vi "MonoVu_exec window.vi"() -> ()   [LabVIEW 2020]
doc: "Sequence Program with the Message Handling Queue (MHQ) for the National High Magnetic Field Laboratory in Tallahassee, Florida. \nOnce you understand how the programs works, you should be able to modify this program easily. If you have any questions, contact Minseong Lee(ml10k@my.fsu.edu), who first made this program in June, 2015."
uses:
  <vilib>/printing/OpenHTMLReport.llb/Open HTML Report in Browser (String).vi
  <vilib>/Utility/NIReport.llb/NI_ReportGenerationCore.lvlib
panel:
  in  "error\ncheck":bool
  out "macro line":i32
  in  "loop stop":bool
  in  "looped command interval (ms)":u32=100
  in  "wait (ms)":u32
  in  "reset error indicator":bool
  out "Error/\nwarning?":bool
  in  "override command error":bool
  in  "platform":u16(ring) items=["Mac", "PC"]
  out "execution count":i32=1
  in  "sequence utility":bool=TRUE caption="seq\n utility"
  out "macro cmd no":i32=34
  in  "go to \ncurrent":bool
  in  "help":bool caption="Help"
  in  "Magnet PS":u16(ring) items=["Resistive Magnet", "SCM2", "SCM1", "Generic SC power supply", "PPMS"]
  out "Buffer Edit":string[](array[string])
  out "Path":path=path "/Users/Shared/NML Data Acquisition/Monovu/sequence templates/SystemABDE_typical.txt"
  out "Buffer History":string[](array[string])
  in  "NML Data Acquisition VI":string(combo)="NML Data Acquisition-New.vi"
  in  "Skip Button":bool caption="Skip"
  out "latest error":errorcluster={"status"=TRUE, "code"=1004, "source"="Open VI Reference in Get_Vi_Data.vi->WaitForAnyVI.vi->MonoVu.vi<APPEND>\nTo load a VI into memory with the Open VI Reference function, a path must be wired for the VI Path input.\n\nVI Name: <b>BLM_ManualControl.vi</b>"}
  in  "error in (no error)":errorcluster
  in  "New Button":bool caption="New"
  in  "Program Stop":bool caption="Program \nStop"
  out "Sequence Status":string="Idle"
  in  "Commands":string(tree)="Set Field"
  in  "Sequence":i32[](listbox)=[19]
  in  "Save Button":bool caption="Save"
  in  "Sequence_Stop":bool caption="Stop"
  in  "Pause Button":bool caption="Pause"
  in  "Run Sequence":bool caption="Run"
  in  "Save As Button":bool caption="Save As"
  out "Cursor Position":i32=19
  out "Current Line":i32
  in  "Open Button":bool caption="Open"
  # "Wait between each execution of command.\ne.g.  if the value is 10, and the command is \n'Wait for Temperature', it checks the temperature every 10 msec. It also forces pause between commands."
  # "(see logbook for previous errors)"
  # "(bypass command syntax error)"
  # "1. Each comand in the sequence line is executed repeatedly until a 'go to next line' command is issued by itself or interrupted by the user. \n2. 'go to next line' condition is defined in the VI for each command. \n\nNote\n(1) For commands with timed or conditioned wait, 'go to next line' command will be issued when the certain condition is met.\n(2) For non-wait command (send command to instruments or VI without waiting response), 'go to next line' is executed automatically.\n(3) For example, 'wait for temperature command' executes repeatedly until the temperature condition is met. The visa reference will be open and closed every time it is executed.\n** Exception: 'Wait for VI value' uses a loop to use the VI reference. The loop condition has to be programmatically reset for the user intervention (skip, pause, stop) accordingly."
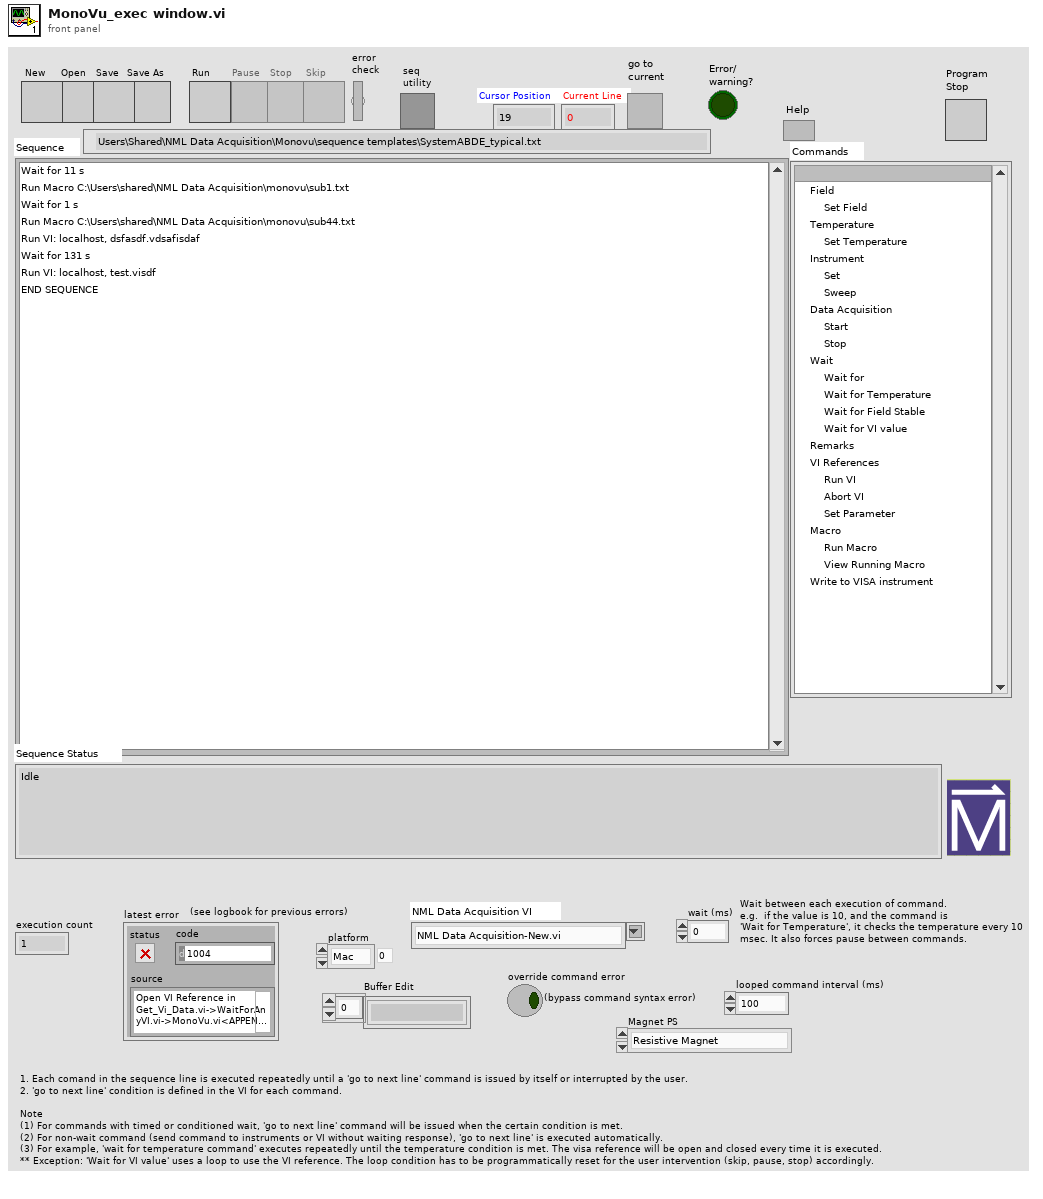
[diagram p1: front panel]
types:
  T1 = cluster{"Sequence_Run":refnum<vi>, "Sequence_Pause":refnum<vi>, "Sequence_Stop":refnum<vi>, "Sequence_Skip":refnum<vi>, "Program Stop":refnum<vi>, "Sequence":refnum<vi>, "NML Data Acquisition VI":refnum<vi>}
  T2 = cluster{"number of line":i32, "Signal":bool, "Command":string, "Sequence Reference":refnum<vi>, "Add or modification":bool}
  T3 = cluster{"No. of command":i32, "Parameters":string[], "Address":refnum<visa-resource-name>, "Boolean":bool, "No. of line":i32, "Initial Time":timestamp, "Current Time":timestamp, "Status":string, "Sequence Ref.":refnum<vi>, "Temp_Check":i32, "Sequence_History":string, "Subsequence":string[]}
  T4 = typedef "Command_Message.ctl" = cluster{"No. of command":i32, "Parameters":string[], "Address":refnum<visa-resource-name>, "Boolean":bool, "No. of line":i32, "Initial Time":timestamp, "Current Time":timestamp, "Status":string, "Sequence Ref.":refnum<vi>, "Temp check":i32, "Sequence_History":string, "Subsequence":string[]}
  T5 = typedef "Button_Reference.ctl" = cluster{"Sequence_Run":refnum<vi>, "Sequence_Pause":refnum<vi>, "Sequence_Stop":refnum<vi>, "Sequence_Skip":refnum<vi>, "Program Stop":refnum<vi>, "Sequence":refnum<vi>, "NML Data Acquisition VI":refnum<vi>}
  T6 = typedef "Command_Queue.ctl" = refnum<queue>
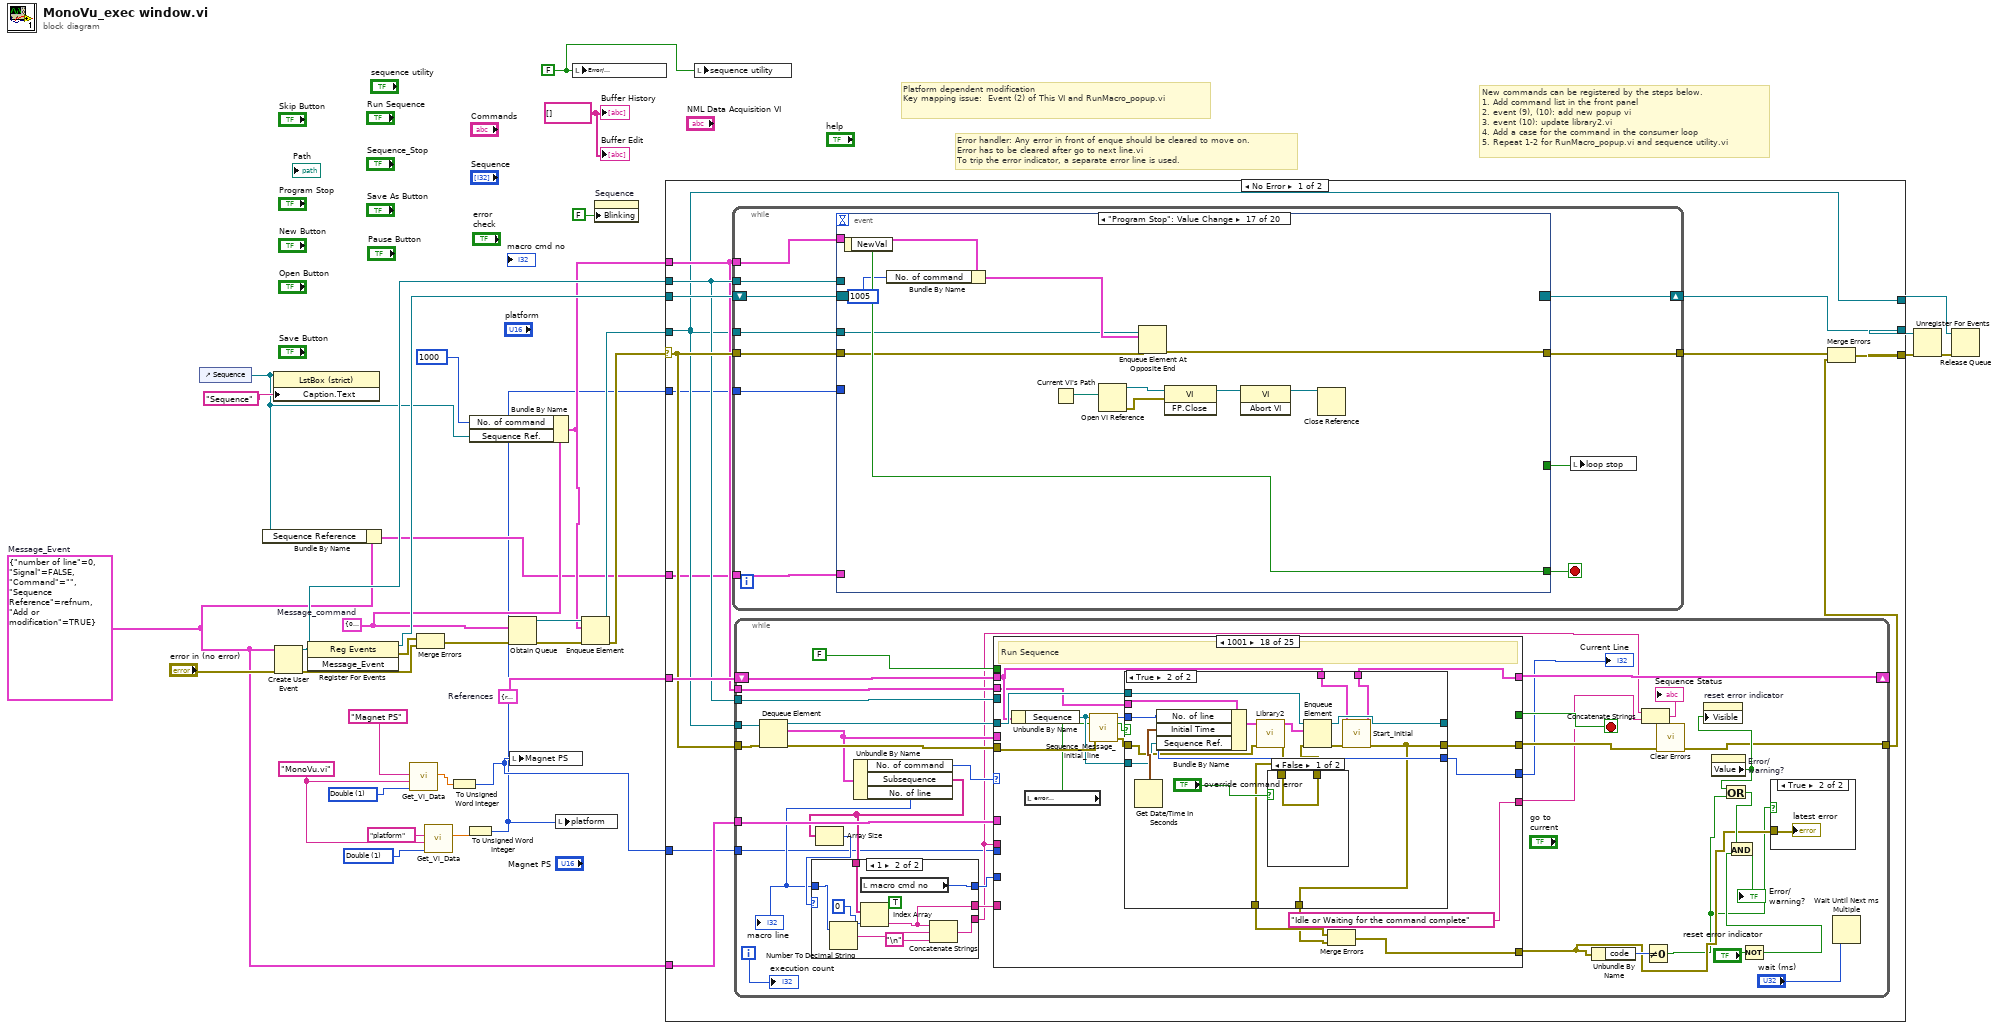
[diagram p0: block diagram]
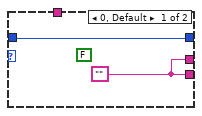
[diagram p3: hidden frame]
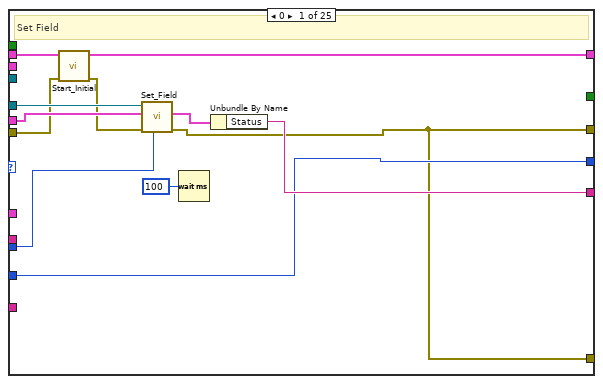
[diagram p4: hidden frame]
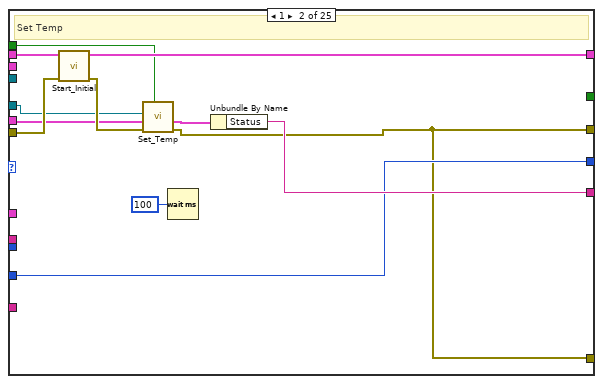
[diagram p5: hidden frame]
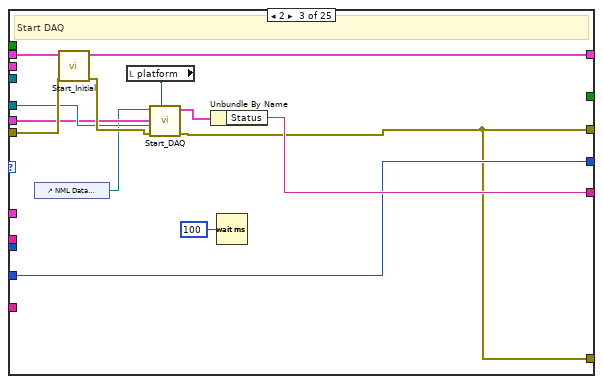
[diagram p6: hidden frame]
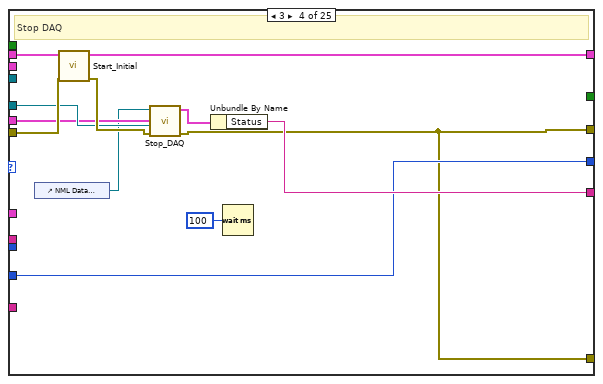
[diagram p7: hidden frame]
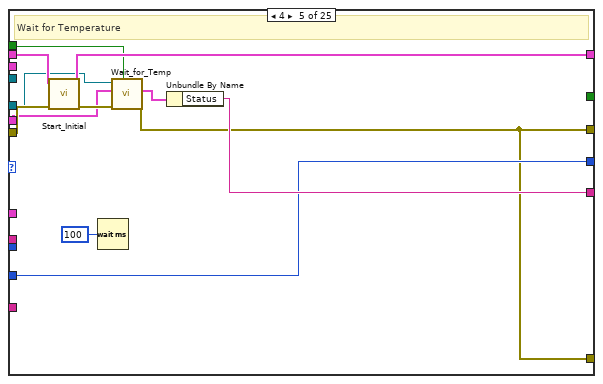
[diagram p8: hidden frame]
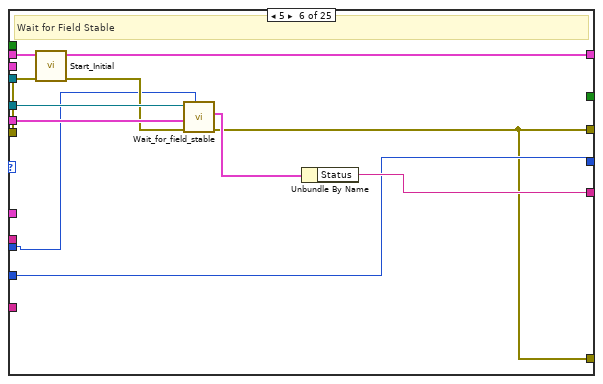
[diagram p9: hidden frame]
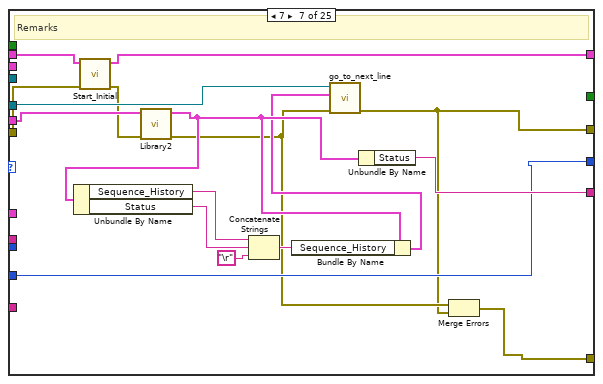
[diagram p10: hidden frame]
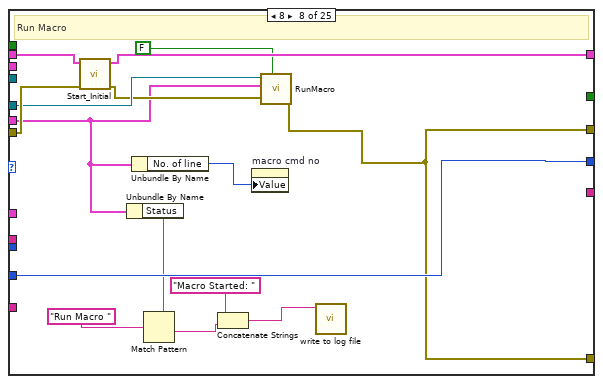
[diagram p11: hidden frame]
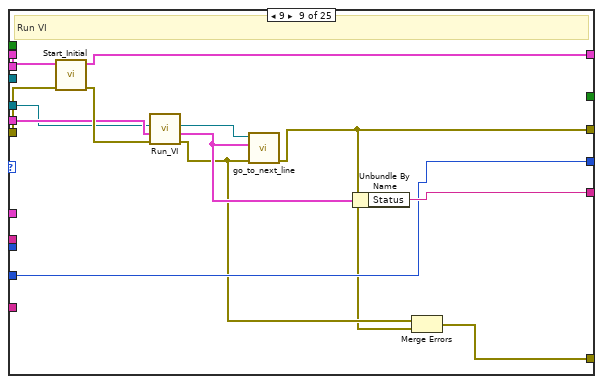
[diagram p12: hidden frame]
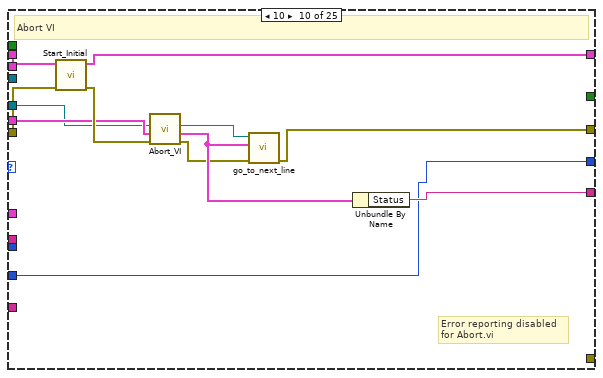
[diagram p13: hidden frame]
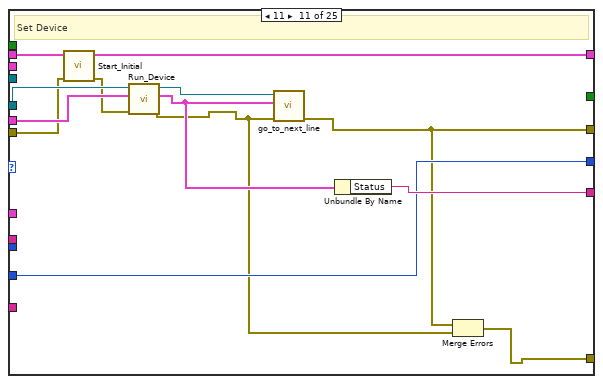
[diagram p14: hidden frame]
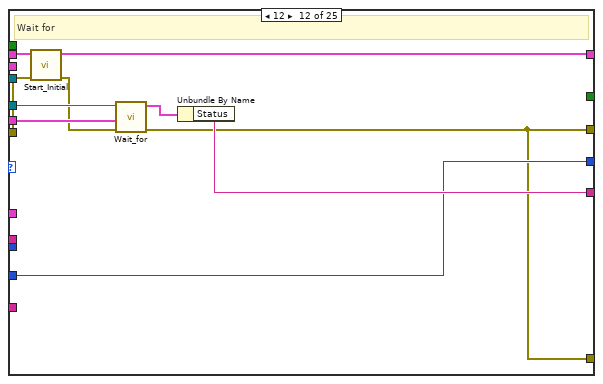
[diagram p15: hidden frame]
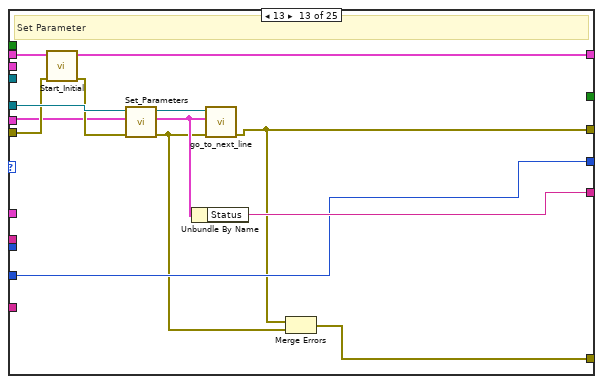
[diagram p16: hidden frame]
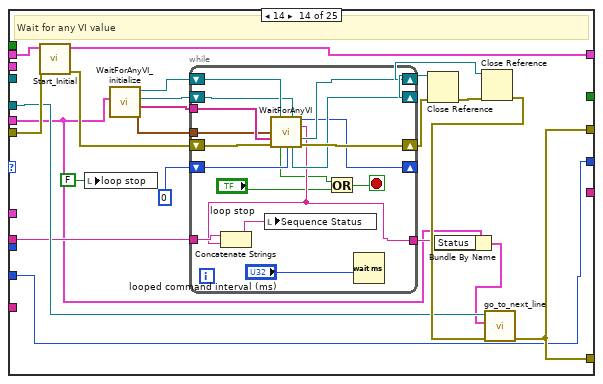
[diagram p17: hidden frame]
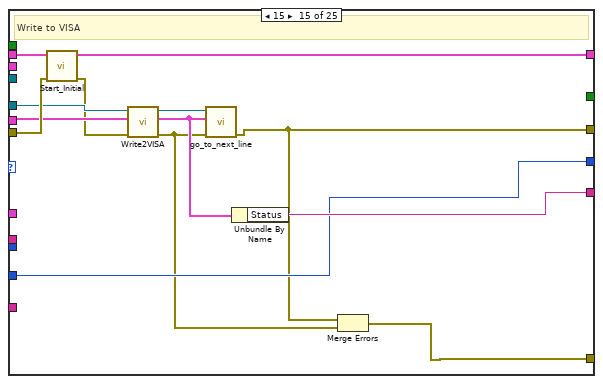
[diagram p18: hidden frame]
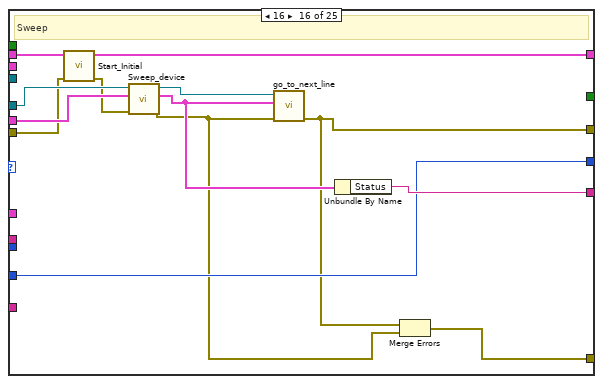
[diagram p19: hidden frame]
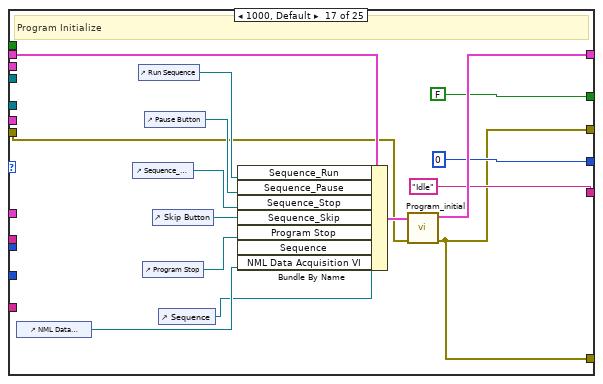
[diagram p20: hidden frame]
diagram:
  w7 = u16 1 items=["String", "Double", "Boolean", "Variant"] ("Data Type")
  w8 = u16 1 items=["String", "Double", "Boolean", "Variant"] ("Data Type")
  w6 = "MonoVu.vi" ("VI Name")
  w10 = FALSE ("Error?")
  w24 = T1 {"Sequence_Run"=refnum, "Sequence_Pause"=refnum, "Sequence_Stop"=refnum, "Sequence_Skip"=refnum, "Program Stop"=refnum, "Sequence"=refnum, "NML Data Acquisition VI"=refnum}  # References
  w12 = string[] []
  w18 = T2 {"number of line"=0, "Signal"=FALSE, "Command"="", "Sequence Reference"=refnum, "Add or modification"=TRUE}  # Message_Event
  w25 = T3 {"No. of command"=0, "Parameters"=[], "Address"="", "Boolean"=TRUE, "No. of line"=0, "Initial Time"=timestamp(0 s since 1904-01-01), "Current Time"=timestamp(0 s since 1904-01-01), "Status"="", "Sequence Ref."=refnum, "Temp_Check"=0, "Sequence_History"="", "Subsequence"=[]}  # Message_command
  # "Error handler: Any error in front of enque should be cleared to move on.\nError has to be cleared after go to next line.vi\nTo trip the error indicator, a separate error line is used."
  # "Platform dependent modification\nKey mapping issue:  Event (2) of This VI and RunMacro_popup.vi"
  # "New commands can be registered by the steps below.\n1. Add command list in the front panel\n2. event (9), (10): add new popup vi\n3. event (10): update library2.vi \n4. Add a case for the command in the consumer loop\n5. Repeat 1-2 for RunMacro_popup.vi and sequence utility.vi"
  n1 = control-ref of="Sequence"() -> (w13:refnum<vi>)
  n2 = Bundle By Name(cluster=w18, "Sequence Reference"=w13) -> (w17:T2)
  n3 = property class="LstBox (strict)"(reference=w13, "Caption.Text"="Sequence") -> ()  [unwired: 1 in, 2 out]
  n4 = Create User Event(user event datatype=w18, error in="error in (no error)") -> (user event=w30:refnum<user-event>, error out=w32:errorcluster)
  n5 = register-events(w30) -> (reference out=w34:refnum<event-registration>, error out=w31:errorcluster)  [unwired: 2 in]
  n6 = call "Get_Vi_Data.vi"("Data Type"=w8, "VI name"=w6, "Control Name"="Magnet PS") -> ("Data (Double)"=w4:dbl)  [unwired: 4 in, 4 out]
  n7 = Merge Errors(w31, w32) -> (w15:errorcluster)
  n8 = call "Get_Vi_Data.vi"("Data Type"=w7, "VI name"=w6, "Control Name"="platform") -> ("Data (Double)"=w3:dbl)  [unwired: 4 in, 4 out]
  n9 = To Unsigned Word Integer(number=w4) -> (unsigned 16bit integer=w2:u16)
  n10 = To Unsigned Word Integer(number=w3) -> (unsigned 16bit integer=w1:u16)
  n11 = Bundle By Name(cluster=w25, "No. of command"=1000, "Sequence Ref."=w13) -> (w23:T3)
  n12 = Obtain Queue(element data type=w25, error in (no error)=w15) -> (queue out=w29:refnum<queue>, error out=w27:errorcluster)  [unwired: 3 in, 1 out]
  n13 = local write "Magnet PS"(w2) -> ()
  n14 = local write "platform"(w1) -> ()
  n15 = local write "Error/\nwarning?"(w10) -> ()
  n16 = Enqueue Element(queue=w29, element=w23, error in (no error)=w27) -> (queue out=w28:refnum<queue>, error out=w26:errorcluster)  [unwired: 1 in, 1 out]
  n17 = property on="Sequence" class="LstBox (strict)"("Blinking"=FALSE) -> ()  [unwired: 2 in, 2 out]
  n18 = case shown="No Error" w26 {
    selector: w26 -> [w45 w1342]
    tunnel: w28 -> [w41 w1340]
    tunnel: [w47 w1342] -> w20
    tunnel: w30 -> [w44 _]
    tunnel: w34 -> [w48 w1341]
    tunnel: w24 -> [w46 _]
    tunnel: w23 -> [w42 _]
    tunnel: w18 -> [w43 _]
    tunnel: [w41 w1340] -> w22
    tunnel: [w39 w1341] -> w21
    tunnel: w17 -> [w37 _]
    tunnel: w1 -> [w36 _]
    tunnel: w2 -> [w35 _]
    frame No Error {
      n19 = while {
        tunnel: w41 -> [w486]
        tunnel: w44 -> [w485]
        tunnel: w45 -> [w484]
        tunnel: [w483] -> w40
        tunnel: w42 -> [w482]
        shift-right: [w481] -> w39
        shift-left: w48 -> [w488]
        tunnel: w37 -> [w480]
        tunnel: w36 -> [w479]
        stop <- w487 stop-if-true
        # "Event_Handler"
        n20 = event shown="[16] \"Program Stop\": Value Change" {
          selector: w488 -> [_ _ _ _ _ _ _ _ _ _ _ _ _ _ _ _ _ _ _ _]
          dyn-events: [_ _ _ _ _ _ _ _ _ _ _ _ _ _ _ _ _ _ _ _] -> w481
          timeout: _ -> [_ _ _ _ _ _ _ _ _ _ _ _ _ _ _ _ _ _ _ _]
          tunnel: [FALSE ("NewVal") FALSE ("NewVal") FALSE ("NewVal") FALSE ("NewVal") FALSE ("NewVal") FALSE ("NewVal") FALSE ("NewVal") FALSE ("NewVal") FALSE ("NewVal") FALSE ("NewVal") FALSE ("NewVal") FALSE ("NewVal") FALSE ("NewVal") FALSE ("NewVal") FALSE ("NewVal") FALSE ("NewVal") w1316 FALSE ("NewVal") TRUE ("NewVal") _] -> w487
          tunnel: w486 -> [w492 _ _ _ _ _ _ _ _ _ _ _ w1253 _ w1290 w1305 w1311 w1319 _ _]
          tunnel: w485 -> [w496 _ w680 w808 _ _ _ _ _ w983 w1112 _ _ _ _ _ _ _ _ _]
          tunnel: w484 -> [w495 w516 w681 w810 w840 w878 w892 w920 w947 w985 w1121 w1242 w1252 _ w1288 w1304 w1312 w1320 w1326 w1335]
          tunnel: [w491 w515 w679 w809 w839 w876 w891 w919 w946 w979 w1108 w1242 w1248 _ w1293 w1300 w1317 w1324 w1326 w1333] -> w483
          tunnel: w482 -> [w493 w514 _ _ _ _ _ _ _ _ w1123 _ w1251 _ w1294 w1303 w1315 w1323 _ _]
          tunnel: w480 -> [_ _ w682 w807 _ _ _ _ _ w977 w1113 _ _ _ _ _ _ _ _ _]
          tunnel: w479 -> [_ _ w676 _ _ _ _ _ _ w981 w1103 _ _ _ _ _ _ _ _ w1338]
          tunnel: [_ _ _ _ _ _ _ _ _ _ _ _ w1246 _ TRUE ("loop stop") TRUE ("loop stop") _ _ _ _] -> w478
          event "Run Sequence": Value Change {
            n21 = event-data() -> ("NewVal"=w494:bool)  [unwired: 1 in]
            n22 = case shown="True" w494 {
              tunnel: w496 -> [_ _]
              tunnel: w495 -> [w497 w501]
              tunnel: w493 -> [_ w504]
              tunnel: w492 -> [w498 w505]
              tunnel: [w498 w500] -> _
              tunnel: [w497 w499] -> w491
              frame False {
              }
              frame True {
                n23 = Bundle By Name(cluster=w504, "No. of command"=1001) -> (w502:T3)
                n24 = Enqueue Element At Opposite End(queue=w505, element=w502, error in (no error)=w501) -> (queue out=w500:refnum<queue>, error out=w499:errorcluster)  [unwired: 1 in, 1 out]
              }
            }
            n25 = call "write to log file.vi"("input"="Run button pressed") -> ()  [unwired: 9 in, 1 out]
          }
          event User Event {
            n26 = event-data() -> ("number of line"=w513:i32, "Command"=w507:string, "Signal"=w511:bool, "Sequence Reference"=w510:refnum<vi>, "Add or modification"=w509:bool)  [unwired: 1 in]
            n27 = local read "Buffer History"() -> (w508:string[])
            n28 = local read "Buffer Edit"() -> (w506:string[])
            n29 = case shown="\"Undo\"" w507 {
              selector: w507 -> [_ _ _ _ _ w632]
              tunnel: w516 -> [w520 w552 w584 w607 w630 w640]
              tunnel: [w518 w543 w575 w603 w616 w639] -> w515
              tunnel: w514 -> [_ _ _ _ _ w638]
              tunnel: w513 -> [_ _ _ _ _ w637]
              tunnel: w511 -> [_ _ _ _ _ w636]
              tunnel: w510 -> [w517 w553 w585 w608 w631 w635]
              tunnel: w509 -> [_ _ _ _ _ w634]
              tunnel: w508 -> [w519 w548 w580 _ w622 w633]
              tunnel: w506 -> [_ _ _ _ w625 _]
              frame "Undo" {
                n30 = Index Array(array=w519, index=0) -> (element=w527:string)
                n31 = Unflatten From String(type=w519, binary string=w527, error in (no error)=w520) -> (value=w526:string[], error out=w525:errorcluster)  [unwired: 2 in, 1 out]
                n32 = property on="Property Node" class="LstBox (strict)"(reference=w517, error in=w525, "Item Names"=w526) -> (error out=w521:errorcluster)  [unwired: 1 out]
                n33 = Delete From Array(array=w519, length=1, index=0) -> (array with subset deleted=w522:string[])  [unwired: 1 out]
                n34 = property on="Buffer History" class="Arr (strict)"(error in=w521, "Val(Sgnl)"=w522) -> (error out=w518:errorcluster)  [unwired: 1 in, 1 out]
              }
              frame "Cut" {
                n35 = property on="Property Node" class="LstBox (strict)"(reference=w553, error in=w552) -> (reference out=w550:refnum<vi>, error out=w549:errorcluster, "Item Names"=w533:string[], "Value"=w529:i32[])
                n36 = Array Size(array=w529) -> (size(s)=w541:i32)
                n37 = Index Array(array=w529, index=0) -> (element=w540:i32)
                n38 = Delete From Array(array=w533, length=w541, index=w540) -> (deleted portion=w531:string[], array with subset deleted=w534:string[])
                n39 = Array Size(array=w531) -> (size(s)=w539:i32)
                n40 = Decrement(x=w539) -> (x-1=w538:i32)
                n41 = Index Array(array=w531, index=w538) -> (element=w536:string)
                n42 = Equal?(x=w536, y="END SEQUENCE") -> (x = y?=w535:bool)
                n43 = case shown="True" w535 {
                  tunnel: w533 -> [_ w561]
                  tunnel: w541 -> [_ w560]
                  tunnel: w540 -> [_ w558]
                  tunnel: [w555 w557] -> w532
                  tunnel: w534 -> [w555 _]
                  tunnel: w531 -> [w554 _]
                  tunnel: [w554 w556] -> w530
                  frame False {
                  }
                  frame True {
                    n44 = Decrement(x=w560) -> (x-1=w559:i32)
                    n45 = Delete From Array(array=w561, length=w559, index=w558) -> (deleted portion=w556:string[], array with subset deleted=w557:string[])
                  }
                }
                n46 = Flatten To String(anything=w532, error in (no error)=w549) -> (data string=w546:string, error out=w545:errorcluster)  [unwired: 2 in, 1 out]
                n47 = property on="Property Node" class="LstBox (strict)"(reference=w550, error in=w545, "Item Names"=w532, "Val(Sgnl)"=w529) -> (error out=w544:errorcluster)  [unwired: 1 out]
                n48 = Insert Into Array(array=w548, index=0, new element=w546) -> (w542:string[])
                n49 = property on="Buffer History" class="Arr (strict)"(error in=w544, "Val(Sgnl)"=w542) -> (error out=w543:errorcluster)  [unwired: 1 in, 1 out]
                n50 = local write "Buffer Edit"(w530) -> ()
              }
              frame "Delete" {
                n51 = property on="Property Node" class="LstBox (strict)"(reference=w585, error in=w584) -> (reference out=w582:refnum<vi>, error out=w581:errorcluster, "Item Names"=w567:string[], "Value"=w562:i32[])
                n52 = Array Size(array=w562) -> (size(s)=w566:i32)
                n53 = Index Array(array=w562, index=0) -> (element=w565:i32)
                n54 = Delete From Array(array=w567, length=w566, index=w565) -> (deleted portion=w573:string[], array with subset deleted=w564:string[])
                n55 = Array Size(array=w573) -> (size(s)=w569:i32)
                n56 = Decrement(x=w569) -> (x-1=w568:i32)
                n57 = Index Array(array=w573, index=w568) -> (element=w572:string)
                n58 = Equal?(x=w572, y="END SEQUENCE") -> (x = y?=w570:bool)
                n59 = case shown="True" w570 {
                  tunnel: w567 -> [_ w591]
                  tunnel: w566 -> [_ w590]
                  tunnel: w565 -> [_ w588]
                  tunnel: [w586 w587] -> w563
                  tunnel: w564 -> [w586 _]
                  frame False {
                  }
                  frame True {
                    n60 = Decrement(x=w590) -> (x-1=w589:i32)
                    n61 = Delete From Array(array=w591, length=w589, index=w588) -> (array with subset deleted=w587:string[])  [unwired: 1 out]
                  }
                }
                n62 = Flatten To String(anything=w563, error in (no error)=w581) -> (data string=w578:string, error out=w577:errorcluster)  [unwired: 2 in, 1 out]
                n63 = property on="Property Node" class="LstBox (strict)"(reference=w582, error in=w577, "Item Names"=w563, "Val(Sgnl)"=w562) -> (error out=w576:errorcluster)  [unwired: 1 out]
                n64 = Insert Into Array(array=w580, index=0, new element=w578) -> (w574:string[])
                n65 = property on="Buffer History" class="Arr (strict)"(error in=w576, "Val(Sgnl)"=w574) -> (error out=w575:errorcluster)  [unwired: 1 in, 1 out]
              }
              frame "Copy" {
                n66 = property on="Property Node" class="LstBox (strict)"(reference=w608, error in=w607) -> (reference out=w605:refnum<vi>, error out=w604:errorcluster, "Item Names"=w593:string[], "Value"=w592:i32[])
                n67 = Array Size(array=w592) -> (size(s)=w597:i32)
                n68 = Index Array(array=w592, index=0) -> (element=w596:i32)
                n69 = Array Subset(array=w593, index=w596, length=w597) -> (w595:string[])
                n70 = Array Size(array=w595) -> (size(s)=w602:i32)
                n71 = Decrement(x=w602) -> (x-1=w601:i32)
                n72 = property on="Property Node" class="LstBox (strict)"(reference=w605, error in=w604, "Item Names"=w593, "Val(Sgnl)"=w592) -> (error out=w603:errorcluster)  [unwired: 1 out]
                n73 = Index Array(array=w595, index=w601) -> (element=w600:string)
                n74 = Equal?(x=w600, y="END SEQUENCE") -> (x = y?=w598:bool)
                n75 = case shown="True" w598 {
                  tunnel: w597 -> [_ w614]
                  tunnel: w596 -> [_ w612]
                  tunnel: [w609 w610] -> w594
                  tunnel: w595 -> [w609 _]
                  tunnel: w593 -> [_ w611]
                  frame False {
                  }
                  frame True {
                    n76 = Decrement(x=w614) -> (x-1=w613:i32)
                    n77 = Delete From Array(array=w611, length=w613, index=w612) -> (deleted portion=w610:string[])  [unwired: 1 out]
                  }
                }
                n78 = local write "Buffer Edit"(w594) -> ()
              }
              frame "Paste" {
                n79 = property on="Property Node" class="LstBox (strict)"(reference=w631, error in=w630) -> (reference out=w628:refnum<vi>, error out=w619:errorcluster, "Item Names"=w626:string[], "Value"=w615:i32[])
                n80 = Index Array(array=w615, index=0) -> (element=w627:i32)
                n81 = Insert Into Array(array=w626, index=w627, new element=w625) -> (w623:string[])
                n82 = Flatten To String(anything=w623, error in (no error)=w619) -> (data string=w624:string, error out=w618:errorcluster)  [unwired: 2 in, 1 out]
                n83 = property on="Property Node" class="LstBox (strict)"(reference=w628, error in=w618, "Item Names"=w623, "Val(Sgnl)"=w615) -> (error out=w617:errorcluster)  [unwired: 1 out]
                n84 = Insert Into Array(array=w622, index=0, new element=w624) -> (w620:string[])
                n85 = property on="Buffer History" class="Arr (strict)"(error in=w617, "Val(Sgnl)"=w620) -> (error out=w616:errorcluster)  [unwired: 1 in, 1 out]
              }
              frame Default {
                n86 = case shown="True" w634 {
                  tunnel: w640 -> [w657 w674]
                  tunnel: [w642 w659] -> w639
                  tunnel: w638 -> [_ _]
                  tunnel: w637 -> [_ _]
                  tunnel: w636 -> [_ _]
                  tunnel: w635 -> [w656 w673]
                  tunnel: w632 -> [w655 w672]
                  tunnel: w633 -> [w654 w671]
                  frame True {
                    n87 = property class="LstBox (strict)"(reference=w656, error in=w657) -> (reference out=w651:refnum<vi>, error out=w646:errorcluster, "Item Names"=w648:string[], "Value"=w641:i32[])
                    n88 = Index Array(array=w641, index=0) -> (element=w652:i32)
                    n89 = Flatten To String(anything=w648, error in (no error)=w646) -> (data string=w649:string, error out=w647:errorcluster)  [unwired: 2 in, 1 out]
                    n90 = Insert Into Array(array=w648, index=w652, new element=w655) -> (w650:string[])
                    n91 = property class="LstBox (strict)"(reference=w651, error in=w647, "Item Names"=w650, "Value"=w641) -> (error out=w643:errorcluster)  [unwired: 1 out]
                    n92 = Insert Into Array(array=w654, index=0, new element=w649) -> (w644:string[])
                    n93 = property on="Buffer History" class="Arr (strict)"(error in=w643, "Val(Sgnl)"=w644) -> (error out=w642:errorcluster)  [unwired: 1 in, 1 out]
                  }
                  frame False {
                    n94 = property class="LstBox (strict)"(reference=w673, error in=w674) -> (reference out=w668:refnum<vi>, error out=w664:errorcluster, "Item Names"=w665:string[], "Value"=w658:i32[])
                    n95 = Index Array(array=w658, index=0) -> (element=w669:i32)
                    n96 = Flatten To String(anything=w665, error in (no error)=w664) -> (data string=w667:string, error out=w663:errorcluster)  [unwired: 2 in, 1 out]
                    n97 = Replace Array Subset(array=w665, new element=w672, index=w669) -> (w666:string[])
                    n98 = property class="LstBox (strict)"(reference=w668, error in=w663, "Item Names"=w666) -> (error out=w661:errorcluster)  [unwired: 1 out]
                    n99 = Insert Into Array(array=w671, index=0, new element=w667) -> (w660:string[])
                    n100 = property on="Buffer History" class="Arr (strict)"(error in=w661, "Val(Sgnl)"=w660) -> (error out=w659:errorcluster)  [unwired: 1 in, 1 out]
                  }
                }
              }
            }
          }
          event "Sequence": Key Down {
            # "PC:\nDelete:  83\nundo: 44\ncut: 45\ncopy: 46\npaste: 47"
            # "Mac:\nDelete:  117\nundo: 6\ncut: 7\ncopy: 8\npaste: 9"
            n101 = event-data() -> ("ScanCode"=w683:i16, "PlatMods.Ctrl"=w677:bool, "PlatMods.Shift"=w675:bool)  [unwired: 1 in]
            n102 = case shown="0, Default" w676 {
              tunnel: w683 -> [w689 w750]
              tunnel: w682 -> [w688 w749]
              tunnel: w681 -> [w687 w748]
              tunnel: w680 -> [w686 w747]
              tunnel: [w685 w746] -> w679
              tunnel: w677 -> [_ w745]
              tunnel: w675 -> [w684 _]
              frame 1 {
                n103 = case shown="0, Default" w689 {
                  tunnel: w688 -> [_ w695 w698 w710 w722 w734]
                  tunnel: w687 -> [w690 w693 w700 w712 w724 w736]
                  tunnel: w686 -> [_ w692 w697 w709 w721 w733]
                  tunnel: [w690 w691 w699 w711 w723 w735] -> w685
                  tunnel: w684 -> [_ _ w701 w713 w725 w737]
                  frame 0, Default {
                  }
                  frame 83 {
                    n104 = Bundle By Name(cluster=w695, "Command"="Delete") -> (w694:T2)
                    n105 = Generate User Event(user event=w692, event data cluster=w694, error in=w693) -> (error out=w691:errorcluster)  [unwired: 1 in, 1 out]
                  }
                  frame 44 {
                    n106 = case shown="True" w701 {
                      tunnel: w700 -> [w702 w704]
                      tunnel: [w702 w706] -> w699
                      tunnel: w698 -> [_ w705]
                      tunnel: w697 -> [_ w703]
                      frame False {
                      }
                      frame True {
                        n107 = Bundle By Name(cluster=w705, "Command"="Undo") -> (w707:T2)
                        n108 = Generate User Event(user event=w703, event data cluster=w707, error in=w704) -> (error out=w706:errorcluster)  [unwired: 1 in, 1 out]
                      }
                    }
                  }
                  frame 45 {
                    n109 = case shown="True" w713 {
                      tunnel: w712 -> [w714 w716]
                      tunnel: [w714 w718] -> w711
                      tunnel: w710 -> [_ w717]
                      tunnel: w709 -> [_ w715]
                      frame False {
                      }
                      frame True {
                        n110 = Bundle By Name(cluster=w717, "Command"="Cut") -> (w719:T2)
                        n111 = Generate User Event(user event=w715, event data cluster=w719, error in=w716) -> (error out=w718:errorcluster)  [unwired: 1 in, 1 out]
                      }
                    }
                  }
                  frame 46 {
                    n112 = case shown="True" w725 {
                      tunnel: w724 -> [w726 w728]
                      tunnel: [w726 w730] -> w723
                      tunnel: w722 -> [_ w729]
                      tunnel: w721 -> [_ w727]
                      frame False {
                      }
                      frame True {
                        n113 = Bundle By Name(cluster=w729, "Command"="Copy") -> (w731:T2)
                        n114 = Generate User Event(user event=w727, event data cluster=w731, error in=w728) -> (error out=w730:errorcluster)  [unwired: 1 in, 1 out]
                      }
                    }
                  }
                  frame 47 {
                    n115 = case shown="True" w737 {
                      tunnel: w736 -> [w738 w740]
                      tunnel: [w738 w742] -> w735
                      tunnel: w734 -> [_ w741]
                      tunnel: w733 -> [_ w739]
                      frame False {
                      }
                      frame True {
                        n116 = Bundle By Name(cluster=w741, "Command"="Paste") -> (w743:T2)
                        n117 = Generate User Event(user event=w739, event data cluster=w743, error in=w740) -> (error out=w742:errorcluster)  [unwired: 1 in, 1 out]
                      }
                    }
                  }
                }
              }
              frame 0, Default {
                n118 = case shown="0, Default" w750 {
                  tunnel: w749 -> [_ w756 w759 w771 w783 w795]
                  tunnel: w748 -> [w751 w754 w761 w773 w785 w797]
                  tunnel: w747 -> [_ w753 w758 w770 w782 w794]
                  tunnel: [w751 w752 w760 w772 w784 w796] -> w746
                  tunnel: w745 -> [_ _ w762 w774 w786 w798]
                  frame 0, Default {
                  }
                  frame 117 {
                    n119 = Bundle By Name(cluster=w756, "Command"="Delete") -> (w755:T2)
                    n120 = Generate User Event(user event=w753, event data cluster=w755, error in=w754) -> (error out=w752:errorcluster)  [unwired: 1 in, 1 out]
                  }
                  frame 6 {
                    n121 = case shown="True" w762 {
                      tunnel: w761 -> [w763 w765]
                      tunnel: [w763 w767] -> w760
                      tunnel: w759 -> [_ w766]
                      tunnel: w758 -> [_ w764]
                      frame False {
                      }
                      frame True {
                        n122 = Bundle By Name(cluster=w766, "Command"="Undo") -> (w768:T2)
                        n123 = Generate User Event(user event=w764, event data cluster=w768, error in=w765) -> (error out=w767:errorcluster)  [unwired: 1 in, 1 out]
                      }
                    }
                  }
                  frame 7 {
                    n124 = case shown="True" w774 {
                      tunnel: w773 -> [w775 w777]
                      tunnel: [w775 w779] -> w772
                      tunnel: w771 -> [_ w778]
                      tunnel: w770 -> [_ w776]
                      frame False {
                      }
                      frame True {
                        n125 = Bundle By Name(cluster=w778, "Command"="Cut") -> (w780:T2)
                        n126 = Generate User Event(user event=w776, event data cluster=w780, error in=w777) -> (error out=w779:errorcluster)  [unwired: 1 in, 1 out]
                      }
                    }
                  }
                  frame 8 {
                    n127 = case shown="True" w786 {
                      tunnel: w785 -> [w787 w789]
                      tunnel: [w787 w791] -> w784
                      tunnel: w783 -> [_ w790]
                      tunnel: w782 -> [_ w788]
                      frame False {
                      }
                      frame True {
                        n128 = Bundle By Name(cluster=w790, "Command"="Copy") -> (w792:T2)
                        n129 = Generate User Event(user event=w788, event data cluster=w792, error in=w789) -> (error out=w791:errorcluster)  [unwired: 1 in, 1 out]
                      }
                    }
                  }
                  frame 9 {
                    n130 = case shown="True" w798 {
                      tunnel: w797 -> [w799 w801]
                      tunnel: [w799 w803] -> w796
                      tunnel: w795 -> [_ w802]
                      tunnel: w794 -> [_ w800]
                      frame False {
                      }
                      frame True {
                        n131 = Bundle By Name(cluster=w802, "Command"="Paste") -> (w804:T2)
                        n132 = Generate User Event(user event=w800, event data cluster=w804, error in=w801) -> (error out=w803:errorcluster)  [unwired: 1 in, 1 out]
                      }
                    }
                  }
                }
              }
            }
          }
          event "Sequence": Shortcut Menu Selection (User) {
            n133 = event-data() -> ("ItemTag"=w811:string)  [unwired: 1 in]
            n134 = case shown="\"Paste\"" w811 {
              selector: w811 -> [_ w816 w822 w828 w834]
              tunnel: w810 -> [w812 w814 w820 w826 w832]
              tunnel: [w812 w813 w819 w825 w831] -> w809
              tunnel: w808 -> [_ w818 w824 w830 w836]
              tunnel: w807 -> [_ w817 w823 w829 w835]
              frame Default {
              }
              frame "Undo" {
                n135 = Bundle By Name(cluster=w817, "Command"=w816) -> (w815:T2)
                n136 = Generate User Event(user event=w818, event data cluster=w815, error in=w814) -> (error out=w813:errorcluster)  [unwired: 1 in, 1 out]
              }
              frame "Cut" {
                n137 = Bundle By Name(cluster=w823, "Command"=w822) -> (w821:T2)
                n138 = Generate User Event(user event=w824, event data cluster=w821, error in=w820) -> (error out=w819:errorcluster)  [unwired: 1 in, 1 out]
              }
              frame "Copy" {
                n139 = Bundle By Name(cluster=w829, "Command"=w828) -> (w827:T2)
                n140 = Generate User Event(user event=w830, event data cluster=w827, error in=w826) -> (error out=w825:errorcluster)  [unwired: 1 in, 1 out]
              }
              frame "Paste" {
                n141 = Bundle By Name(cluster=w835, "Command"=w834) -> (w833:T2)
                n142 = Generate User Event(user event=w836, event data cluster=w833, error in=w832) -> (error out=w831:errorcluster)  [unwired: 1 in, 1 out]
              }
            }
          }
          event "New Button": Value Change {
            n143 = event-data() -> ("NewVal"=w841:bool, "CtlRef"=w838:refnum<vi>)  [unwired: 1 in]
            n144 = case shown="True" w841 {
              tunnel: w840 -> [w842 w858]
              tunnel: [w842 w850] -> w839
              tunnel: w838 -> [_ w853]
              frame False {
              }
              frame True {
                n145 = property on="Sequence" class="LstBox (strict)"(error in=w858) -> (error out=w849:errorcluster, "Caption.Text"=w857:string, "Item Names"=w854:string[])  [unwired: 1 in, 1 out]
                n146 = property on="Buffer History" class="Arr (strict)"(error in=w849) -> (error out=w848:errorcluster, "Value"=w847:string[])  [unwired: 1 in, 1 out]
                n147 = Equal?(x=w857, y="Sequence*") -> (x = y?=w855:bool)
                n148 = case shown="False" w855 {
                  tunnel: w848 -> [w863 w874]
                  tunnel: w854 -> [_ w875]
                  tunnel: [w864 w869] -> w846
                  tunnel: w853 -> [w862 w868]
                  tunnel: [w862 w868] -> w852
                  tunnel: w847 -> [_ w866]
                  tunnel: [string[] [] ("Buffer out") w865] -> w844
                  frame False {
                    n149 = property on="Sequence" class="LstBox (strict)"(error in=w863, "Item Names"=string[] ["END SEQUENCE"], "Caption.Text"="Sequence") -> (error out=w864:errorcluster)  [unwired: 1 in, 1 out]
                  }
                  frame True {
                    n150 = property on="Path" class="Path"(error in=w874) -> (error out=w873:errorcluster, "Value"=w872:path)  [unwired: 1 in, 1 out]
                    n151 = call "New_File.vi"("error in (no error)"=w873, "Path"=w872, "Buffer in"=w866, "Sequence in"=w875) -> ("error out"=w871:errorcluster, "Sequence Caption"=w867:string, "Buffer out"=w865:string[], "Sequence_out"=w870:string[])  [unwired: 4 in]
                    n152 = property on="Sequence" class="LstBox (strict)"(error in=w871, "Item Names"=w870, "Caption.Text"=w867) -> (error out=w869:errorcluster)  [unwired: 1 in, 1 out]
                  }
                }
                n153 = property on="Buffer History" class="Arr (strict)"(error in=w846, "Value"=w844) -> (error out=w845:errorcluster)  [unwired: 1 in, 1 out]
                n154 = property class="Bool (strict)"(reference=w852, error in=w845, "Value"=FALSE) -> (error out=w850:errorcluster)  [unwired: 1 out]
                n155 = property on="Sequence" class="LstBox (strict)"("Top Row"=0) -> ()  [unwired: 2 in, 2 out]
              }
            }
          }
          event "Buffer History": Value Change {
            n156 = event-data() -> ("NewVal"=w882:string[])  [unwired: 1 in]
            n157 = Array Size(array=w882) -> (size(s)=w881:i32)
            n158 = Equal?(x=w881, y=0) -> (x = y?=w879:bool)
            n159 = case shown="False" w879 {
              tunnel: w878 -> [w884 w887]
              tunnel: [w883 w886] -> w876
              frame True {
                n160 = property on="Sequence" class="LstBox (strict)"(error in=w884, "Caption.Text"="Sequence") -> (error out=w883:errorcluster)  [unwired: 1 in, 1 out]
              }
              frame False {
                n161 = property on="Sequence" class="LstBox (strict)"(error in=w887, "Caption.Text"="Sequence*") -> (error out=w886:errorcluster)  [unwired: 1 in, 1 out]
              }
            }
          }
          event "Open Button": Value Change {
            n162 = event-data() -> ("NewVal"=w893:bool, "CtlRef"=w890:refnum<vi>)  [unwired: 1 in]
            n163 = case shown="True" w893 {
              tunnel: w892 -> [w894 w916]
              tunnel: [w894 w897] -> w891
              tunnel: w890 -> [_ w900]
              frame False {
              }
              frame True {
                n164 = property on="Sequence" class="LstBox (strict)"(error in=w916) -> (error out=w912:errorcluster, "Caption.Text"=w914:string, "Item Names"=w913:string[])  [unwired: 1 in, 1 out]
                n165 = Equal?(x=w914, y="Sequence*") -> (x = y?=w901:bool)
                n166 = property on="Buffer History" class="Arr (strict)"(error in=w912) -> (error out=w910:errorcluster, "Value"=w911:string[])  [unwired: 1 in, 1 out]
                n167 = property on="Path" class="Path"(error in=w910) -> (error out=w908:errorcluster, "Value"=w909:path)  [unwired: 1 in, 1 out]
                n168 = call "Open_File.vi"("Message?"=w901, "Path in"=w909, "error in (no error)"=w908, "Sequence in"=w913, "Buffer in"=w911, "Sequence Caption in"=w914) -> ("error out"=w896:errorcluster, "Sequence out"=w906:string[], "Buffer out"=w904:string[], "Sequence Caption out"=w907:string, "Path out"=w902:path, "top row"=w895:i32)
                n169 = property on="Sequence" class="LstBox (strict)"("Top Row"=w895) -> ()  [unwired: 2 in, 2 out]
                n170 = property on="Sequence" class="LstBox (strict)"(error in=w896, "Item Names"=w906, "Caption.Text"=w907) -> (error out=w905:errorcluster)  [unwired: 1 in, 1 out]
                n171 = property on="Buffer History" class="Arr (strict)"(error in=w905, "Value"=w904) -> (error out=w903:errorcluster)  [unwired: 1 in, 1 out]
                n172 = property on="Path" class="Path"(error in=w903, "Value"=w902) -> (error out=w899:errorcluster)  [unwired: 1 in, 1 out]
                n173 = property class="Bool (strict)"(reference=w900, error in=w899, "Value"=FALSE) -> (error out=w897:errorcluster)  [unwired: 1 out]
              }
            }
          }
          event "Save Button": Value Change {
            n174 = event-data() -> ("NewVal"=w921:bool, "CtlRef"=w918:refnum<vi>)  [unwired: 1 in]
            n175 = case shown="True" w921 {
              tunnel: w920 -> [w922 w939]
              tunnel: [w922 w923] -> w919
              tunnel: w918 -> [_ w926]
              frame False {
              }
              frame True {
                n176 = property on="Path" class="Path"(error in=w939) -> (error out=w938:errorcluster, "Value"=w941:path)  [unwired: 1 in, 1 out]
                n177 = Not Equal?(x=path "", y=w941) -> (x != y?=w942:bool)
                n178 = property on="Buffer History" class="Arr (strict)"(error in=w938) -> (error out=w937:errorcluster, "Value"=w940:string[])  [unwired: 1 in, 1 out]
                n179 = property on="Sequence" class="LstBox (strict)"(error in=w937) -> (error out=w936:errorcluster, "Item Names"=w935:string[], "Caption.Text"=w934:string)  [unwired: 1 in, 1 out]
                n180 = call "Save_File.vi"("Sequence caption in"=w934, "Path?"=w942, "error in (no error)"=w936, "Sequence in"=w935, "Buffer in"=w940, "Path in"=w941) -> ("error out"=w933:errorcluster, "Sequence out"=w929:string[], "Buffer out"=w931:string[], "Path out"=w927:path, "Sequence caption out"=w930:string)  [unwired: 1 in]
                n181 = property on="Buffer History" class="Arr (strict)"(error in=w933, "Value"=w931) -> (error out=w932:errorcluster)  [unwired: 1 in, 1 out]
                n182 = property on="Sequence" class="LstBox (strict)"(error in=w932, "Item Names"=w929, "Caption.Text"=w930) -> (error out=w928:errorcluster)  [unwired: 1 in, 1 out]
                n183 = property on="Path" class="Path"(error in=w928, "Value"=w927) -> (error out=w925:errorcluster)  [unwired: 1 in, 1 out]
                n184 = property class="Bool (strict)"(reference=w926, error in=w925, "Value"=FALSE) -> (error out=w923:errorcluster)  [unwired: 1 out]
              }
            }
          }
          event "Save As Button": Value Change {
            n185 = event-data() -> ("NewVal"=w948:bool, "CtlRef"=w945:refnum<vi>)  [unwired: 1 in]
            n186 = case shown="True" w948 {
              tunnel: w947 -> [w949 w967]
              tunnel: [w949 w951] -> w946
              tunnel: w945 -> [_ w954]
              frame False {
              }
              frame True {
                n187 = property on="Path" class="Path"(error in=w967) -> (error out=w966:errorcluster, "Value"=w969:path)  [unwired: 1 in, 1 out]
                n188 = property on="Buffer History" class="Arr (strict)"(error in=w966) -> (error out=w965:errorcluster, "Value"=w968:string[])  [unwired: 1 in, 1 out]
                n189 = property on="Sequence" class="LstBox (strict)"(error in=w965) -> (error out=w964:errorcluster, "Item Names"=w963:string[], "Caption.Text"=w962:string)  [unwired: 1 in, 1 out]
                n190 = call "Save_File.vi"("Sequence caption in"=w962, "Path?"=FALSE, "error in (no error)"=w964, "Sequence in"=w963, "Buffer in"=w968, "Path in"=w969) -> ("error out"=w961:errorcluster, "Sequence out"=w957:string[], "Buffer out"=w959:string[], "Path out"=w955:path, "Sequence caption out"=w958:string)  [unwired: 1 in]
                n191 = property on="Buffer History" class="Arr (strict)"(error in=w961, "Value"=w959) -> (error out=w960:errorcluster)  [unwired: 1 in, 1 out]
                n192 = property on="Sequence" class="LstBox (strict)"(error in=w960, "Item Names"=w957, "Caption.Text"=w958) -> (error out=w956:errorcluster)  [unwired: 1 in, 1 out]
                n193 = property on="Path" class="Path"(error in=w956, "Value"=w955) -> (error out=w953:errorcluster)  [unwired: 1 in, 1 out]
                n194 = property class="Bool (strict)"(reference=w954, error in=w953, "Value"=FALSE) -> (error out=w951:errorcluster)  [unwired: 1 out]
              }
            }
          }
          event "Commands": Double Click {
            n195 = event-data() -> ("Tag"=w984:string)  [unwired: 1 in]
            n196 = case shown="\"Run VI\"" w984 {
              tunnel: w985 -> [w996 w1002 w1008 w1014 w1020 w1026 w1032 w1038 w1044 w1050 w1056 w1062 w1065 w1070 w1078 w1086 w1087 w1092]
              tunnel: [w996 w1000 w1005 w1012 w1017 w1023 w1029 w1035 w1041 w1047 w1053 w1059 w1065 w1070 w1075 w1081 w1089 w1095] -> w980
              tunnel: w983 -> [w995 w999 w1006 w1013 w1019 w1025 w1031 w1037 w1043 w1049 w1055 w1061 w1067 w1072 w1077 w1083 _ w1097]
              tunnel: w981 -> [_ _ _ _ _ _ _ _ _ _ _ _ _ _ _ w1084 _ _]
              tunnel: [TRUE ("Cancel") w1001 w1007 w1011 w1018 w1024 w1030 w1036 w1042 w1048 w1054 w1060 FALSE ("Signal") FALSE ("Signal") w1076 w1082 _ w1096] -> w972
              tunnel: [w995 w999 w1006 w1013 w1019 w1025 w1031 w1037 w1043 w1049 w1055 w1061 w1067 w1072 w1077 w1083 _ w1097] -> w978
              tunnel: [_ TRUE ("Add or modification") TRUE ("Add or modification") TRUE ("Add or modification") TRUE ("Add or modification") TRUE ("Add or modification") TRUE ("Add or modification") TRUE ("Add or modification") TRUE ("Add or modification") TRUE ("Add or modification") TRUE ("Add or modification") TRUE ("Add or modification") TRUE ("Add or modification") TRUE ("Add or modification") TRUE ("Signal") TRUE ("Signal") _ TRUE ("Add or modification")] -> w976
              tunnel: [_ w998 w1003 w1009 w1015 w1021 w1027 w1033 w1039 w1046 w1051 w1057 "Stop" ("Command") "Wait for Field Stable" ("Command") w1073 w1079 _ w1093] -> w974
              frame Default {
              }
              frame "Set Field" {
                n197 = call "SetField_popup.vi"("error in (no error)"=w1002) -> ("Output Line command"=w998:string, "Cancel"=w1001:bool, "error out"=w1000:errorcluster)  [unwired: 5 in]
              }
              frame "Set Temperature" {
                n198 = call "SetTemp_popup.vi"("error in (no error)"=w1008) -> ("error out"=w1005:errorcluster, "Cancel"=w1007:bool, "Output Line Command"=w1003:string)  [unwired: 7 in]
              }
              frame "Wait for Temperature" {
                n199 = call "SetWaitForTemp_popup.vi"("error in (no error)"=w1014) -> ("Output Line Command"=w1009:string, "Cancel"=w1011:bool, "error out"=w1012:errorcluster)  [unwired: 7 in]
              }
              frame "Wait for" {
                n200 = call "SetWaitFor_popup.vi"("error in (no error)"=w1020) -> ("error out"=w1017:errorcluster, "Cancel"=w1018:bool, "Output Line Command"=w1015:string)  [unwired: 7 in]
              }
              frame "Start" {
                n201 = call "SetStart_popup.vi"("error in (no error)"=w1026) -> ("Output Line Command"=w1021:string, "Cancel"=w1024:bool, "error out"=w1023:errorcluster)  [unwired: 7 in]
              }
              frame "Remarks" {
                n202 = call "SetRemarks_popup.vi"("error in (no error)"=w1032) -> ("Cancel"=w1030:bool, "Output Line Command"=w1027:string, "error out"=w1029:errorcluster)  [unwired: 7 in]
              }
              frame "Run VI" {
                n203 = call "SetRunVI_popup.vi"("error in (no error)"=w1038) -> ("Cancel"=w1036:bool, "Output Line Command"=w1033:string, "error out"=w1035:errorcluster)  [unwired: 7 in]
              }
              frame "Abort VI" {
                n204 = call "SetAbortVI_popup.vi"("error in (no error)"=w1044) -> ("Cancel"=w1042:bool, "Output Line Command"=w1039:string, "error out"=w1041:errorcluster)  [unwired: 7 in]
              }
              frame "Set Parameter" {
                n205 = call "SetParameter_popup.vi"("error in (no error)"=w1050) -> ("error out"=w1047:errorcluster, "Cancel"=w1048:bool, "Output Line Command"=w1046:string)  [unwired: 7 in]
              }
              frame "Set" {
                n206 = call "SetDevice_popup.vi"("error in (no error)"=w1056) -> ("Cancel"=w1054:bool, "Output Line Command"=w1051:string, "error out"=w1053:errorcluster)  [unwired: 7 in]
              }
              frame "Sweep" {
                n207 = call "SetSweep_popup.vi"("error in (no error)"=w1062) -> ("Cancel"=w1060:bool, "Output Line Command"=w1057:string, "error out"=w1059:errorcluster)  [unwired: 7 in]
              }
              frame "Stop" {
              }
              frame "Wait for Field Stable" {
              }
              frame "Wait for VI value" {
                n208 = call "SetWaitForAnyVI_popup.vi"("error in (no error)"=w1078) -> ("error out"=w1075:errorcluster, "Cancel"=w1076:bool, "Output Line Command"=w1073:string)  [unwired: 7 in]
              }
              frame "Run Macro" {
                n209 = call "RunMacro_popup.vi"("load?"=FALSE, "platform"=w1084, "error in (no error)"=w1086) -> ("Cancel"=w1082:bool, "command out"=w1079:string, "error out"=w1081:errorcluster)  [unwired: 5 in]
              }
              frame "View Running Macro" {
                n210 = vi-ref "RunMacro.vi"() -> (w1091:refnum<vi>)
                n211 = invoke class="VI" method="FP.Open"(reference=w1091, error in=w1087) -> (reference out=w1090:refnum<vi>, error out=w1088:errorcluster)  [unwired: 3 in, 3 out]
                n212 = Close Reference(reference=w1090, error in (no error)=w1088) -> (error out=w1089:errorcluster)
              }
              frame "Write to VISA instrument" {
                n213 = call "WriteVISA_popup.vi"("error in (no error)"=w1092) -> ("Output Line Command"=w1093:string, "Cancel"=w1096:bool, "error out"=w1095:errorcluster)  [unwired: 8 in]
              }
            }
            n214 = local read "error\ncheck"() -> (w970:bool)
            n215 = case shown="True" w970 {
              tunnel: w974 -> [_ w989]
              tunnel: [FALSE ("error") w987] -> w973
              frame False {
              }
              frame True {
                n216 = Build Array(w989) -> (w988:string[])
                n217 = call "sequence util_error check.vi"("Item Names IN"=w988) -> ("error"=w987:bool)  [unwired: 8 in, 1 out]
              }
            }
            n218 = Or(x=w972, y=w973) -> (x .or. y?=w971:bool)
            n219 = Bundle By Name(cluster=w977, "Signal"=w972, "Command"=w974, "Add or modification"=w976) -> (w975:T2)
            n220 = case shown="False" w971 {
              tunnel: w978 -> [w992 _]
              tunnel: w975 -> [w991 _]
              tunnel: [w990 w993] -> w979
              tunnel: w980 -> [_ w993]
              frame False {
                n221 = Generate User Event(user event=w992, event data cluster=w991) -> (error out=w990:errorcluster)  [unwired: 2 in, 1 out]
              }
              frame True {
              }
            }
          }
          event "Sequence": Double Click {
            # "check if the sequence is changed. Returns 'False\"\nIf (1) 'cancel' button pressed \nOR (2) 'ok' button pressed but no value change"
            n222 = event-data() -> ("Row"=w1114:i32)  [unwired: 1 in]
            n223 = Bundle By Name(cluster=w1123, "No. of line"=w1114) -> (w1122:T3)
            n224 = Unbundle By Name(w1113) -> ("Sequence Reference"=w1118:refnum<vi>)
            n225 = call "Library2.vi"("Message_command_in"=w1122, "error in (no error)"=w1121) -> ("Message_command out"=w1120:T4, "error out"=w1117:errorcluster)  [unwired: 7 in]
            n226 = property class="LstBox (strict)"(reference=w1118, error in=w1117) -> (error out=w1116:errorcluster, "Item Names"=w1115:string[])  [unwired: 1 out]
            n227 = Unbundle By Name(w1120) -> ("No. of command"=w1119:i32)
            n228 = local read "error\ncheck"() -> (w1098:bool)
            n229 = Index Array(array=w1115, index=w1114) -> (element=w1104:string)
            n230 = case shown="13" w1119 {
              tunnel: w1116 -> [w1143 w1150 w1157 w1164 w1171 w1178 w1187 w1194 w1201 w1208 w1215 w1222 w1223 w1236 w1240]
              tunnel: w1104 -> [w1142 w1149 w1156 w1163 w1170 w1173 w1186 w1193 w1200 w1207 w1214 w1221 w1227 w1235 _]
              tunnel: w1113 -> [w1140 w1147 w1154 w1161 w1168 w1180 w1184 w1191 w1198 w1205 w1212 w1219 w1229 w1233 w1239]
              tunnel: w1112 -> [w1139 w1146 w1153 w1160 w1167 w1179 w1183 w1190 w1197 w1204 w1211 w1218 w1228 w1232 w1238]
              tunnel: [w1141 w1148 w1155 w1162 w1169 w1175 w1185 w1192 w1199 w1206 w1213 w1216 w1226 w1234 w1240] -> w1109
              tunnel: [w1140 w1147 w1154 w1161 w1168 w1180 w1184 w1191 w1198 w1205 w1212 w1219 w1229 w1233 w1239] -> w1111
              tunnel: [w1139 w1146 w1153 w1160 w1167 w1179 w1183 w1190 w1197 w1204 w1211 w1218 w1228 w1232 w1238] -> w1110
              tunnel: [w1138 w1145 w1152 w1159 w1166 w1176 w1182 w1189 w1196 w1202 w1209 w1217 w1225 w1231 TRUE ("Cancel")] -> w1105
              tunnel: [w1137 w1144 w1151 w1158 w1165 w1177 w1181 w1188 w1195 w1203 w1210 w1220 w1224 w1230 _] -> w1101
              tunnel: w1103 -> [_ _ _ _ _ w1172 _ _ _ _ _ _ _ _ _]
              frame 0 {
                n231 = call "SetField_popup.vi"("error in (no error)"=w1143, "Input Line command"=w1142) -> ("Output Line command"=w1137:string, "Cancel"=w1138:bool, "error out"=w1141:errorcluster)  [unwired: 4 in]
              }
              frame 1 {
                n232 = call "SetTemp_popup.vi"("Input Line Command"=w1149, "error in (no error)"=w1150) -> ("error out"=w1148:errorcluster, "Cancel"=w1145:bool, "Output Line Command"=w1144:string)  [unwired: 6 in]
              }
              frame 2 {
                n233 = call "SetStart_popup.vi"("Input Line Command"=w1156, "error in (no error)"=w1157) -> ("Output Line Command"=w1151:string, "Cancel"=w1152:bool, "error out"=w1155:errorcluster)  [unwired: 6 in]
              }
              frame 4 {
                n234 = call "SetWaitForTemp_popup.vi"("Input Line Command"=w1163, "error in (no error)"=w1164) -> ("Output Line Command"=w1158:string, "Cancel"=w1159:bool, "error out"=w1162:errorcluster)  [unwired: 6 in]
              }
              frame 7 {
                n235 = call "SetRemarks_popup.vi"("Input Line Command"=w1170, "error in (no error)"=w1171) -> ("Cancel"=w1166:bool, "Output Line Command"=w1165:string, "error out"=w1169:errorcluster)  [unwired: 6 in]
              }
              frame 8 {
                n236 = call "RunMacro_popup.vi"("load?"=TRUE, "platform"=w1172, "command in"=w1173, "error in (no error)"=w1178) -> ("Cancel"=w1176:bool, "command out"=w1177:string, "error out"=w1175:errorcluster)  [unwired: 4 in]
              }
              frame 9 {
                n237 = call "SetRunVI_popup.vi"("Input Line Command"=w1186, "error in (no error)"=w1187) -> ("Cancel"=w1182:bool, "Output Line Command"=w1181:string, "error out"=w1185:errorcluster)  [unwired: 6 in]
              }
              frame 10 {
                n238 = call "SetAbortVI_popup.vi"("Input Line Command"=w1193, "error in (no error)"=w1194) -> ("Cancel"=w1189:bool, "Output Line Command"=w1188:string, "error out"=w1192:errorcluster)  [unwired: 6 in]
              }
              frame 11 {
                n239 = call "SetDevice_popup.vi"("Input Line Command"=w1200, "error in (no error)"=w1201) -> ("Cancel"=w1196:bool, "Output Line Command"=w1195:string, "error out"=w1199:errorcluster)  [unwired: 6 in]
              }
              frame 12 {
                n240 = call "SetWaitFor_popup.vi"("Input Line Command"=w1207, "error in (no error)"=w1208) -> ("error out"=w1206:errorcluster, "Cancel"=w1202:bool, "Output Line Command"=w1203:string)  [unwired: 6 in]
              }
              frame 13 {
                n241 = call "SetParameter_popup.vi"("Input Line Command"=w1214, "error in (no error)"=w1215) -> ("error out"=w1213:errorcluster, "Cancel"=w1209:bool, "Output Line Command"=w1210:string)  [unwired: 6 in]
              }
              frame 14 {
                n242 = call "SetWaitForAnyVI_popup.vi"("Input Line Command"=w1221, "error in (no error)"=w1222) -> ("error out"=w1216:errorcluster, "Cancel"=w1217:bool, "Output Line Command"=w1220:string)  [unwired: 6 in]
              }
              frame 15 {
                n243 = call "WriteVISA_popup.vi"("error in (no error)"=w1223, "Input Line Command"=w1227) -> ("Output Line Command"=w1224:string, "Cancel"=w1225:bool, "error out"=w1226:errorcluster)  [unwired: 7 in]
              }
              frame 16 {
                n244 = call "SetSweep_popup.vi"("Input Line Command"=w1235, "error in (no error)"=w1236) -> ("Cancel"=w1231:bool, "Output Line Command"=w1230:string, "error out"=w1234:errorcluster)  [unwired: 6 in]
              }
              frame Default {
              }
            }
            n245 = case shown="False" w1098 {
              tunnel: w1101 -> [_ w1127]
              tunnel: [FALSE ("error") w1125] -> w1102
              frame False {
              }
              frame True {
                n246 = Build Array(w1127) -> (w1126:string[])
                n247 = call "sequence util_error check.vi"("Item Names IN"=w1126) -> ("error"=w1125:bool)  [unwired: 8 in, 1 out]
              }
            }
            n248 = Equal?(x=w1104, y=w1101) -> (x = y?=w1106:bool)
            n249 = Or(x=w1105, y=w1106) -> (x .or. y?=w1100:bool)
            n250 = Or(x=w1100, y=w1102) -> (x .or. y?=w1099:bool)
            n251 = case shown="True" w1099 {
              selector: w1099 -> [w1130 _]
              tunnel: w1111 -> [w1134 _]
              tunnel: w1110 -> [w1132 _]
              tunnel: w1101 -> [w1131 _]
              tunnel: w1109 -> [w1129 w1136]
              tunnel: [w1128 w1136] -> w1108
              frame False {
                n252 = Bundle By Name(cluster=w1134, "Signal"=w1130, "Command"=w1131, "Add or modification"=FALSE) -> (w1133:T2)
                n253 = Generate User Event(user event=w1132, event data cluster=w1133, error in=w1129) -> (error out=w1128:errorcluster)  [unwired: 1 in, 1 out]
              }
              frame True {
              }
            }
          }
          event "Sequence": Value Change {
            n254 = event-data() -> ("NewVal"=w1245:i32[])  [unwired: 1 in]
            n255 = Index Array(array=w1245, index=0) -> (element=→"Cursor Position":i32)
          }
          event "Pause Button": Value Change {
            # "Note: unpause restart the execution line. For example, if it was paused\nduring 'Wait for 1 hr' line, the stopwatch will reset after unpause (waiting\nanother 1 hr). \nFor the subsequence, it restarts the line of the subsequence."
            # "for the looped command, \npause will stop the loop,\nunpause will resume the loop"
            n256 = event-data() -> ("NewVal"=w1250:bool)  [unwired: 1 in]
            n257 = local read "Current Line"() -> (w1249:i32)
            n258 = case shown="True" w1250 {
              tunnel: w1253 -> [w1260 w1270]
              tunnel: w1252 -> [_ w1269]
              tunnel: w1251 -> [w1256 w1268]
              tunnel: w1250 -> [_ w1266]
              tunnel: w1249 -> [w1259 w1265]
              tunnel: [w1258 w1262] -> w1248
              tunnel: [FALSE ("loop stop") TRUE ("loop stop")] -> w1246
              frame False {
                n259 = Decrement(x=w1259) -> (x-1=w1257:i32)
                n260 = Bundle By Name(cluster=w1256, "No. of line"=w1257) -> (w1255:T3)
                n261 = call "go_to_next_line.vi"("Message_command in"=w1255, "Command Queue in"=w1260) -> ("error out"=w1258:errorcluster)  [unwired: 8 in, 1 out]
              }
              frame True {
                n262 = flat-sequence {
                  frame #0 {
                    w1273 = "RunMacro.vi" ("VI Name")
                    n263 = local read "macro line"() -> (w1271:i32)
                    n264 = call "set_control_in_Memory.vi"("Control Name"="restart line", "Value"=w1271, "VI Name"=w1273) -> ()  [unwired: 2 in, 1 out]
                    n265 = call "set_control_in_Memory.vi"("Control Name"="paused?", "Value"=TRUE ("loop stop"), "VI Name"=w1273) -> ()  [unwired: 2 in, 1 out]
                  }
                }
                n266 = Bundle By Name(cluster=w1268, "No. of command"=1002, "Boolean"=w1266, "No. of line"=w1265, "Status"="Pause" ("Sequence status")) -> (w1264:T3)
                n267 = Enqueue Element At Opposite End(queue=w1270, element=w1264, error in (no error)=w1269) -> (error out=w1262:errorcluster)  [unwired: 1 in, 2 out]
              }
            }
          }
          event "go to \ncurrent": Value Change {
            w1282 = 10  # halfline
            n268 = event-data() -> ()  [unwired: 1 in, 1 out]
            n269 = local read "Current Line"() -> (w1283:i32)
            n270 = local read "Sequence"() -> (w1281:i32[])
            n271 = Subtract(x=w1283, y=w1282) -> (x-y=w1277:i32)
            n272 = Replace Array Subset(array=w1281, new element=w1283, index=0) -> (w1279:i32[])
            n273 = local write "Sequence"(w1279) -> ()
            n274 = Max & Min(x=u8 0, y=w1277) -> (max(x,y)=w1276:i32)  [unwired: 1 out]
            n275 = property on="Sequence" class="LstBox (strict)"("Top Row"=w1276) -> ()  [unwired: 2 in, 2 out]
          }
          event "Skip Button": Value Change {
            n276 = event-data() -> ()  [unwired: 1 in, 1 out]
            n277 = Bundle By Name(cluster=w1294, "No. of command"=1004) -> (w1291:T3)
            n278 = Flush Queue(queue=w1290, error in (no error)=w1288) -> (queue out=w1289:refnum<queue>, error out=w1287:errorcluster)  [unwired: 1 out]
            n279 = Enqueue Element At Opposite End(queue=w1289, element=w1291, error in (no error)=w1287) -> (error out=w1293:errorcluster)  [unwired: 1 in, 2 out]
          }
          event "Sequence_Stop": Value Change {
            n280 = event-data() -> ("NewVal"=w1302:bool)  [unwired: 1 in]
            n281 = local read "Current Line"() -> (w1301:i32)
            n282 = Bundle By Name(cluster=w1303, "No. of command"=1003, "Boolean"=w1302, "No. of line"=w1301, "Status"="Pause" ("Sequence status")) -> (w1298:T3)
            n283 = Enqueue Element At Opposite End(queue=w1305, element=w1298, error in (no error)=w1304) -> (error out=w1300:errorcluster)  [unwired: 1 in, 2 out]
          }
          event "Program Stop": Value Change {
            n284 = event-data() -> ("NewVal"=w1316:bool)  [unwired: 1 in]
            n285 = Bundle By Name(cluster=w1315, "No. of command"=1005) -> (w1313:T3)
            n286 = Current VI's Path() -> (path=w1309:path)
            n287 = Open VI Reference(vi path=w1309) -> (vi reference=w1308:refnum<vi>, error out=w1310:errorcluster)  [unwired: 5 in]
            n288 = Enqueue Element At Opposite End(queue=w1311, element=w1313, error in (no error)=w1312) -> (error out=w1317:errorcluster)  [unwired: 1 in, 2 out]
            n289 = invoke class="VI" method="FP.Close"(reference=w1308, error in=w1310) -> (reference out=w1307:refnum<vi>)  [unwired: 1 in, 2 out]
            n290 = invoke class="VI" method="Abort VI"(reference=w1307) -> (reference out=w1306:refnum<vi>)  [unwired: 2 in, 2 out]
            n291 = Close Reference(reference=w1306) -> ()  [unwired: 1 in, 1 out]
          }
          event "help": Value Change {
            n292 = event-data() -> ()  [unwired: 1 in, 1 out]
            n293 = Bundle By Name(cluster=w1323, "No. of command"=1006) -> (w1321:T3)
            n294 = Enqueue Element At Opposite End(queue=w1319, element=w1321, error in (no error)=w1320) -> (error out=w1324:errorcluster)  [unwired: 1 in, 2 out]
          }
          event Application Instance Close? {
            n295 = event-data() -> ()  [unwired: 1 in, 5 out]
            n296 = event-data("SilentShutdown"=TRUE) -> ()  [unwired: 1 in, 1 out]
          }
          event "sequence utility": Value Change {
            # "If true, current sequence and file path will be exported."
            n297 = event-data() -> ("CtlRef"=w1336:refnum<vi>)  [unwired: 1 in, 5 out]
            n298 = property on="Sequence" class="LstBox (strict)"() -> ("Item Names"=w1330:string[])  [unwired: 2 in, 2 out]
            n299 = property class="Bool (strict)"(reference=w1336, error in=w1335, "Value"=FALSE) -> (error out=w1334:errorcluster)  [unwired: 1 out]
            n300 = local read "Path"() -> (w1331:path)
            n301 = call "sequence utility.vi"("sequence in"=w1330, "error in (no error)"=w1334, "sequence path"=w1331, "platform"=w1338, "export?"=TRUE) -> ("error out"=w1333:errorcluster, "changed sequence"=w1328:string[], "do not update seq."=w1329:bool)  [unwired: 4 in]
            n302 = case shown="False" w1329 {
              tunnel: w1328 -> [w1339 _]
              frame False {
                n303 = property on="Sequence" class="LstBox (strict)"("Item Names"=w1339) -> ()  [unwired: 2 in, 2 out]
              }
              frame True {
              }
            }
          }
        }
        n304 = local write "loop stop"(w478) -> ()
      }
      n305 = while {
        shift-right: [w77] -> _
        shift-left: w46 -> [w78]
        tunnel: w41 -> [w76]
        tunnel: w45 -> [w75]
        tunnel: w44 -> [w74]
        tunnel: [w57] -> w38
        tunnel: w43 -> [w68]
        tunnel: w42 -> [w72]
        tunnel: w35 -> [w49]
        i -> [w64]
        stop <- w83 stop-if-true
        # "Message_Handler"
        n306 = Dequeue Element(queue=w76, error in (no error)=w75) -> (queue out=w81:refnum<queue>, element=w80:T3, error out=w82:errorcluster)  [unwired: 1 in, 1 out]
        n307 = Unbundle By Name(w80) -> ("No. of command"=w79:i32, "Subsequence"=w67:string[], "No. of line"=w50:i32)
        "macro line" <- w50
        n308 = Array Size(array=w67) -> (size(s)=w69:i32)
        n309 = case shown="1" w69 {
          tunnel: w67 -> [_ w94]
          tunnel: [w85 w89] -> w51
          tunnel: [w86 w92] -> w65
          tunnel: w50 -> [w86 w88]
          tunnel: [w85 w87] -> w53
          frame 0, Default {
            (unwired) FALSE ("Visible")
            w85 = ""
          }
          frame 1 {
            (unwired) TRUE ("Visible")
            n310 = Number To Decimal String(number=w88) -> (decimal integer string=w90:string)  [unwired: 1 in]
            n311 = local read "macro cmd no"() -> (w92:i32)
            n312 = Index Array(array=w94, index=0) -> (element=w87:string)
            n313 = Concatenate Strings(w87, w90, "\n") -> (w89:string)
          }
        }
        n314 = case shown="1001" w79 {
          tunnel: [_ _ _ _ _ _ _ _ _ _ _ _ _ _ _ _ FALSE _ _ _ _ TRUE _ _ _] -> w83
          tunnel: w82 -> [w101 w116 w129 w141 w153 w165 w181 w197 w209 w221 w232 w242 w256 w279 w309 w320 w328 w355 w389 w404 w427 w434 _ w455 w476]
          tunnel: [w95 w107 w119 w132 w144 w156 w168 w190 w200 w212 w225 w237 w247 w266 w299 w313 w325 w345 w385 w395 w408 w434 _ w446 w469] -> w73
          tunnel: w80 -> [w106 w110 w125 w137 w148 w162 w179 w187 w207 w219 w233 w245 w254 w261 w305 w321 _ _ _ _ w414 _ _ _ w473]
          tunnel: w81 -> [w105 w113 w126 w138 w152 w163 w182 w195 w206 w218 w234 w246 w257 w267 w306 w322 _ w353 w390 w405 w428 _ _ w466 w474]
          tunnel: w78 -> [w102 w117 w130 w142 w155 w166 w183 w198 w211 w223 w236 w240 w259 w281 w311 w324 w339 w348 w394 w402 w431 w435 w441 w456 w477]
          tunnel: [w99 w114 w128 w140 w154 w164 w180 w196 w210 w222 w235 w239 w258 w280 w310 w323 w331 w347 w393 w403 w430 w435 w441 w457 w475] -> w77
          tunnel: w74 -> [_ _ _ _ _ _ _ _ _ _ _ _ _ _ _ _ _ _ _ _ _ _ _ _ _]
          tunnel: w68 -> [_ _ _ _ _ _ _ _ _ _ _ _ _ _ _ _ _ _ _ _ _ _ _ _ _]
          tunnel: w72 -> [_ _ _ _ _ _ _ _ _ _ _ _ _ _ _ _ _ w341 _ _ _ _ _ w452 _]
          tunnel: [w96 w108 w121 w133 w145 w157 w170 w192 w202 w214 w227 w238 w250 w265 w307 w315 0 ("No. of line") w346 w391 w406 w422 0 ("No. of line") _ _ w471] -> w71
          tunnel: [w103 w118 w131 w143 w149 w159 w177 _ w203 w215 w229 w243 w251 _ w308 w317 "Idle" ("Status") "Idle or Waiting for the command complete" ("Status") "Pause" ("Status") "Idle" ("Status") "Skip" ("Sequence status") "Program Close" ("Sequence status") _ _ _] -> w70
          tunnel: FALSE ("Use LS336Panel.vi") -> [_ w109 _ _ w146 _ _ _ _ _ _ _ _ _ _ _ _ _ _ _ _ _ _ _ _]
          tunnel: w49 -> [w97 _ _ _ _ w158 _ _ _ _ _ _ _ _ _ _ _ _ _ _ _ _ _ _ _]
          tunnel: w65 -> [w96 w108 w121 w133 w145 w157 w170 w192 w202 w214 w227 w238 w250 w265 w307 w315 _ _ _ _ _ _ _ _ w471]
          tunnel: [w95 w107 w119 w132 w144 w156 w167 w190 w199 _ w224 w237 w249 w266 w301 w312 w325 w342 w385 w395 w408 w434 errorcluster {"status"=FALSE, "code"=0, "source"=""} ("error out") w445 w469] -> w55
          tunnel: w53 -> [_ _ _ _ _ _ _ _ _ _ _ _ _ _ _ _ _ _ _ _ _ _ _ w444 _]
          tunnel: w51 -> [_ _ _ _ _ _ _ _ _ _ _ _ _ w264 _ _ _ _ _ _ _ _ _ _ _]
          frame 0 {
            # "Set Field"
            n315 = call "Start_Initial.vi"("error in (no error)"=w101, "Reference"=w102) -> ("error out"=w100:errorcluster, "dup Reference"=w99:T5)  [unwired: 8 in]
            n316 = call "Set_Field.vi"("Magnet PS"=w97, "error in (no error)"=w100, "Command_message_in"=w106, "Command_queue_in"=w105) -> ("error out"=w95:errorcluster, "Command_message_out"=w104:T4)  [unwired: 5 in, 1 out]
            n317 = Wait (ms)(milliseconds to wait=u32 100) -> ()  [unwired: 1 out]
            n318 = Unbundle By Name(w104) -> ("Status"=w103:string)
          }
          frame 1 {
            # "Set Temp"
            n319 = call "Start_Initial.vi"("error in (no error)"=w116, "Reference"=w117) -> ("error out"=w115:errorcluster, "dup Reference"=w114:T5)  [unwired: 8 in]
            n320 = call "Set_Temp.vi"("LS336FrontPanel.vi"=w109, "error in (no error)"=w115, "Message_command_in"=w110, "Command_queue_in"=w113) -> ("error out"=w107:errorcluster, "Message_command_out"=w112:T4)  [unwired: 6 in]
            n321 = Wait (ms)(milliseconds to wait=u32 100) -> ()  [unwired: 1 out]
            n322 = Unbundle By Name(w112) -> ("Status"=w118:string)
          }
          frame 2 {
            # "Start DAQ"
            n323 = control-ref of="NML Data Acquisition VI"() -> (w123:refnum<vi>)
            n324 = call "Start_Initial.vi"("error in (no error)"=w129, "Reference"=w130) -> ("error out"=w127:errorcluster, "dup Reference"=w128:T5)  [unwired: 8 in]
            n325 = local read "platform"() -> (w120:u16)
            n326 = call "Start_DAQ.vi"("platform"=w120, "error in (no error)"=w127, "Command_Queue_in"=w126, "Command_message_in"=w125, "DAQ in"=w123) -> ("error out"=w119:errorcluster, "Command_message_out"=w124:T4)  [unwired: 5 in]
            n327 = Unbundle By Name(w124) -> ("Status"=w131:string)
            n328 = Wait (ms)(milliseconds to wait=u32 100) -> ()  [unwired: 1 out]
          }
          frame 3 {
            # "Stop DAQ"
            n329 = control-ref of="NML Data Acquisition VI"() -> (w135:refnum<vi>)
            n330 = call "Start_Initial.vi"("error in (no error)"=w141, "Reference"=w142) -> ("error out"=w139:errorcluster, "dup Reference"=w140:T5)  [unwired: 8 in]
            n331 = call "Stop_DAQ.vi"("error in (no error)"=w139, "Command_Queue_in"=w138, "Command_message_in"=w137, "DAQ in"=w135) -> ("error out"=w132:errorcluster, "Command_message_out"=w136:T4)  [unwired: 6 in]
            n332 = Unbundle By Name(w136) -> ("Status"=w143:string)
            n333 = Wait (ms)(milliseconds to wait=u32 100) -> ()  [unwired: 1 out]
          }
          frame 4 {
            # "Wait for Temperature"
            n334 = call "Start_Initial.vi"("error in (no error)"=w153, "Reference"=w155) -> ("error out"=w151:errorcluster, "dup Reference"=w154:T5)  [unwired: 8 in]
            n335 = Wait (ms)(milliseconds to wait=u32 100) -> ()  [unwired: 1 out]
            n336 = call "Wait_for_Temp.vi"("LS336FrontPanel.vi"=w146, "error in (no error)"=w151, "Message_command in"=w148, "Command Queue"=w152) -> ("error out"=w144:errorcluster, "dup Message_command"=w150:T4)  [unwired: 6 in]
            n337 = Unbundle By Name(w150) -> ("Status"=w149:string)
          }
          frame 5 {
            # "Wait for Field Stable"
            n338 = call "Start_Initial.vi"("error in (no error)"=w165, "Reference"=w166) -> ("error out"=w161:errorcluster, "dup Reference"=w164:T5)  [unwired: 8 in]
            n339 = call "Wait_for_field_stable.vi"("Magnet PS"=w158, "error in (no error)"=w161, "Message_command in"=w162, "Command_Queue"=w163) -> ("error out"=w156:errorcluster, "Message_command out"=w160:T4)  [unwired: 6 in]
            n340 = Unbundle By Name(w160) -> ("Status"=w159:string)
          }
          frame 7 {
            # "Remarks"
            n341 = call "Start_Initial.vi"("error in (no error)"=w181, "Reference"=w183) -> ("error out"=w178:errorcluster, "dup Reference"=w180:T5)  [unwired: 8 in]
            n342 = call "Library2.vi"("Message_command_in"=w179, "error in (no error)"=w178) -> ("Message_command out"=w172:T4, "error out"=w169:errorcluster)  [unwired: 7 in]
            n343 = Unbundle By Name(w172) -> ("Sequence_History"=w176:string, "Status"=w175:string)
            n344 = Concatenate Strings(w176, w175, "\r") -> (w173:string)
            n345 = Bundle By Name(cluster=w172, "Sequence_History"=w173) -> (w171:T4)
            n346 = call "go_to_next_line.vi"("error in (no error)"=w169, "Message_command in"=w171, "Command Queue in"=w182) -> ("error out"=w168:errorcluster)  [unwired: 7 in, 1 out]
            n347 = Unbundle By Name(w172) -> ("Status"=w177:string)
            n348 = Merge Errors(w169, w168) -> (w167:errorcluster)
          }
          frame 8 {
            # "Run Macro"
            n349 = call "Start_Initial.vi"("error in (no error)"=w197, "Reference"=w198) -> ("error out"=w194:errorcluster, "dup Reference"=w196:T5)  [unwired: 8 in]
            n350 = Unbundle By Name(w187) -> ("Status"=w186:string)
            n351 = Unbundle By Name(w187) -> ("No. of line"=w193:i32)
            n352 = Match Pattern(string=w186, regular expression="Run Macro ") -> (after substring=w184:string)  [unwired: 1 in, 3 out]
            n353 = Concatenate Strings("Macro Started: " ("input"), w184) -> (w188:string)
            n354 = property on="macro cmd no" class="DigNum (strict)"("Value"=w193) -> ()  [unwired: 2 in, 2 out]
            n355 = call "RunMacro.vi"("submacro"=FALSE, "error in (no error)"=w194, "Message_command"=w187, "queue"=w195) -> ("error out"=w190:errorcluster)  [unwired: 5 in, 2 out]
            n356 = call "write to log file.vi"("input"=w188) -> ()  [unwired: 9 in, 1 out]
          }
          frame 9 {
            # "Run VI"
            n357 = call "Start_Initial.vi"("error in (no error)"=w209, "Reference"=w211) -> ("error out"=w208:errorcluster, "dup Reference"=w210:T5)  [unwired: 8 in]
            n358 = call "Run_VI.vi"("error in (no error)"=w208, "Message_command_in"=w207, "Command Queue in"=w206) -> ("error out"=w201:errorcluster, "Message_command out"=w204:T4, "Command Queue out"=w205:T6)  [unwired: 5 in, 1 out]
            n359 = call "go_to_next_line.vi"("error in (no error)"=w201, "Message_command in"=w204, "Command Queue in"=w205) -> ("error out"=w200:errorcluster)  [unwired: 7 in, 1 out]
            n360 = Unbundle By Name(w204) -> ("Status"=w203:string)
            n361 = Merge Errors(w201, w200) -> (w199:errorcluster)
          }
          frame 10 {
            # "Error reporting disabled\nfor Abort.vi"
            # "Abort VI"
            n362 = call "Start_Initial.vi"("error in (no error)"=w221, "Reference"=w223) -> ("error out"=w220:errorcluster, "dup Reference"=w222:T5)  [unwired: 8 in]
            n363 = call "Abort_VI.vi"("error in (no error)"=w220, "Message_command_in"=w219, "Command Queue in"=w218) -> ("error out"=w213:errorcluster, "Message_command out"=w216:T4, "Command Queue out"=w217:T6)  [unwired: 5 in, 1 out]
            n364 = call "go_to_next_line.vi"("error in (no error)"=w213, "Message_command in"=w216, "Command Queue in"=w217) -> ("error out"=w212:errorcluster)  [unwired: 7 in, 1 out]
            n365 = Unbundle By Name(w216) -> ("Status"=w215:string)
          }
          frame 11 {
            # "Set Device"
            n366 = call "Start_Initial.vi"("error in (no error)"=w232, "Reference"=w236) -> ("error out"=w231:errorcluster, "dup Reference"=w235:T5)  [unwired: 8 in]
            n367 = call "Run_Device.vi"("error in (no error)"=w231, "Message_command"=w233, "Command Queue"=w234) -> ("error out"=w226:errorcluster, "dup Message_command"=w228:T4, "dup Command Queue"=w230:T6)  [unwired: 6 in]
            n368 = call "go_to_next_line.vi"("error in (no error)"=w226, "Message_command in"=w228, "Command Queue in"=w230) -> ("error out"=w225:errorcluster)  [unwired: 7 in, 1 out]
            n369 = Unbundle By Name(w228) -> ("Status"=w229:string)
            n370 = Merge Errors(w225, w226) -> (w224:errorcluster)
          }
          frame 12 {
            # "Wait for"
            n371 = call "Start_Initial.vi"("error in (no error)"=w242, "Reference"=w240) -> ("error out"=w241:errorcluster, "dup Reference"=w239:T5)  [unwired: 8 in]
            n372 = call "Wait_for.vi"("error in (no error)"=w241, "Message_command in"=w245, "Command Queue"=w246) -> ("error out"=w237:errorcluster, "dup Message_command"=w244:T4)  [unwired: 7 in]
            n373 = Unbundle By Name(w244) -> ("Status"=w243:string)
          }
          frame 13 {
            # "Set Parameter"
            n374 = call "Start_Initial.vi"("error in (no error)"=w256, "Reference"=w259) -> ("error out"=w255:errorcluster, "dup Reference"=w258:T5)  [unwired: 8 in]
            n375 = call "Set_Parameters.vi"("error in (no error)"=w255, "Message_command In"=w254, "Command Queue In"=w257) -> ("error out"=w248:errorcluster, "Message_command Out"=w252:T4, "Command Queue out"=w253:T6)  [unwired: 6 in]
            n376 = Unbundle By Name(w252) -> ("Status"=w251:string)
            n377 = call "go_to_next_line.vi"("error in (no error)"=w248, "Message_command in"=w252, "Command Queue in"=w253) -> ("error out"=w247:errorcluster)  [unwired: 7 in, 1 out]
            n378 = Merge Errors(w247, w248) -> (w249:errorcluster)
          }
          frame 14 {
            # "Wait for any VI value"
            n379 = call "Start_Initial.vi"("error in (no error)"=w279, "Reference"=w281) -> ("error out"=w278:errorcluster, "dup Reference"=w280:T5)  [unwired: 8 in]
            n380 = local write "loop stop"(FALSE ("loop stop")) -> ()
            n381 = call "WaitForAnyVI_initialize.vi"("Message_command In"=w261) -> ("current time"=w270:timestamp, "parameters"=w272:string[], "vi reference"=w276:refnum<vi>, "application reference"=w277:refnum<vi>)  [unwired: 7 in]
            n382 = while {
              shift-right: [w297] -> w269
              shift-left: w278 -> [w298]
              shift-right: [w296] -> w273
              shift-left: w277 -> [w293]
              shift-right: [w295] -> w274
              shift-left: w276 -> [w292]
              tunnel: w272 -> [w294]
              shift-right: [w289] -> _
              shift-left: u32 0 ("millisecond timer value") -> [w291]
              tunnel: w270 -> [w290]
              tunnel: w264 -> [w288]
              tunnel: [w286] -> w262
              stop <- w284 stop-if-true
              n383 = call "WaitForAnyVI.vi"("application reference"=w293, "vi reference"=w292, "Initial Time"=w290, "parameters"=w294, "error in (no error)"=w298, "counter in"=w291) -> ("counter out"=w289:i32, "status"=w286:string, "application reference out"=w296:refnum<vi>, "Done"=w283:bool, "vi reference out"=w295:refnum<vi>, "error out"=w297:errorcluster)  [unwired: 4 in]
              n384 = Concatenate Strings(w288, w286) -> (w287:string)
              n385 = local write "Sequence Status"(w287) -> ()
              n386 = Or(x=w283, y="loop stop") -> (x .or. y?=w284:bool)
              n387 = Wait (ms)(milliseconds to wait="looped command interval (ms)") -> ()  [unwired: 1 out]
            }
            n388 = Close Reference(reference=w274, error in (no error)=w269) -> (error out=w275:errorcluster)
            n389 = Bundle By Name(cluster=w261, "Status"=w262) -> (w263:T3)
            n390 = Close Reference(reference=w273, error in (no error)=w275) -> (error out=w268:errorcluster)
            n391 = call "go_to_next_line.vi"("error in (no error)"=w268, "Message_command in"=w263, "Command Queue in"=w267) -> ("error out"=w266:errorcluster)  [unwired: 7 in, 1 out]
          }
          frame 15 {
            # "Write to VISA"
            n392 = call "Start_Initial.vi"("error in (no error)"=w309, "Reference"=w311) -> ("error out"=w304:errorcluster, "dup Reference"=w310:T5)  [unwired: 8 in]
            n393 = call "Write2VISA.vi"("error in (no error)"=w304, "Message_command In"=w305, "Command Queue In"=w306) -> ("error out"=w300:errorcluster, "Message_command Out"=w302:T4, "Command Queue out"=w303:T6)  [unwired: 6 in]
            n394 = call "go_to_next_line.vi"("error in (no error)"=w300, "Message_command in"=w302, "Command Queue in"=w303) -> ("error out"=w299:errorcluster)  [unwired: 7 in, 1 out]
            n395 = Unbundle By Name(w302) -> ("Status"=w308:string)
            n396 = Merge Errors(w299, w300) -> (w301:errorcluster)
          }
          frame 16 {
            # "Sweep"
            n397 = call "Start_Initial.vi"("error in (no error)"=w320, "Reference"=w324) -> ("error out"=w319:errorcluster, "dup Reference"=w323:T5)  [unwired: 8 in]
            n398 = call "Sweep_device.vi"("error in (no error)"=w319, "Message_command"=w321, "Command Queue"=w322) -> ("error out"=w314:errorcluster, "dup Message_command"=w316:T4, "dup Command Queue"=w318:T6)  [unwired: 6 in]
            n399 = call "go_to_next_line.vi"("error in (no error)"=w314, "Message_command in"=w316, "Command Queue in"=w318) -> ("error out"=w313:errorcluster)  [unwired: 7 in, 1 out]
            n400 = Unbundle By Name(w316) -> ("Status"=w317:string)
            n401 = Merge Errors(w313, w314) -> (w312:errorcluster)
          }
          frame 1000, Default {
            # "Program Initialize"
            n402 = control-ref of="NML Data Acquisition VI"() -> (w333:refnum<vi>)
            n403 = control-ref of="Sequence_Stop"() -> (w336:refnum<vi>)
            n404 = control-ref of="Run Sequence"() -> (w338:refnum<vi>)
            n405 = control-ref of="Program Stop"() -> (w334:refnum<vi>)
            n406 = control-ref of="Pause Button"() -> (w337:refnum<vi>)
            n407 = control-ref of="Skip Button"() -> (w335:refnum<vi>)
            n408 = control-ref of="Sequence"() -> (w326:refnum<vi>)
            n409 = Bundle By Name(cluster=w339, "Sequence_Run"=w338, "Sequence_Pause"=w337, "Sequence_Stop"=w336, "Sequence_Skip"=w335, "Program Stop"=w334, "Sequence"=w326, "NML Data Acquisition VI"=w333) -> (w332:T5)
            n410 = call "Program_initial.vi"("error in (no error)"=w328, "Reference"=w332) -> ("error out"=w325:errorcluster, "dup Reference"=w331:T5)  [unwired: 8 in]
          }
          frame 1001 {
            # "Run Sequence"
            n411 = Unbundle By Name(w348) -> ("Sequence"=w350:refnum<vi>)
            n412 = local read "error\ncheck"() -> (w340:bool)
            n413 = call "Sequence_Message_initial_line.vi"("reference"=w350, "error check?"=w340, "error in (no error)"=w355) -> ("Number of begin"=w351:u16, "Run?"=w354:bool, "error out"=w352:errorcluster)  [unwired: 5 in]
            n414 = case shown="True" w354 {
              tunnel: w353 -> [w366 w379]
              tunnel: w352 -> [w357 w371]
              tunnel: [w356 w367] -> w345
              tunnel: w341 -> [w359 w382]
              tunnel: w351 -> [_ w372]
              tunnel: [w362 w378] -> _
              tunnel: w350 -> [_ w376]
              tunnel: w348 -> [w365 w375]
              tunnel: [w365 w373] -> w347
              tunnel: [w358 w372] -> w346
              tunnel: [w357 w368] -> w344
              tunnel: [w356 w367] -> w343
              frame False {
                n415 = Unbundle By Name(w359) -> ("No. of line"=w358:i32)
                n416 = Bundle By Name(cluster=w359, "No. of command"=1000, "No. of line"=w358) -> (w360:T3)
                n417 = Flush Queue(queue=w366, error in (no error)=w357) -> (queue out=w364:refnum<queue>, error out=w363:errorcluster)  [unwired: 1 out]
                n418 = Enqueue Element(queue=w364, element=w360, error in (no error)=w363) -> (queue out=w362:refnum<queue>, error out=w356:errorcluster)  [unwired: 1 in, 1 out]
              }
              frame True {
                n419 = Get Date/Time In Seconds() -> (seconds since 1Jan1904=w377:timestamp)
                n420 = Bundle By Name(cluster=w382, "No. of line"=w372, "Initial Time"=w377, "Sequence Ref."=w376) -> (w381:T3)
                n421 = call "Library2.vi"("Message_command_in"=w381, "error in (no error)"=w371) -> ("Message_command out"=w380:T4, "error out"=w368:errorcluster)  [unwired: 7 in]
                n422 = case shown="False" "override command error" {
                  tunnel: [w383 errorcluster {"status"=FALSE, "code"=0, "source"=""} ("error in (no error)")] -> w369
                  tunnel: w368 -> [w383 _]
                  frame False {
                  }
                  frame True {
                  }
                }
                n423 = Enqueue Element(queue=w379, element=w380, error in (no error)=w369) -> (queue out=w378:refnum<queue>, error out=w374:errorcluster)  [unwired: 1 in, 1 out]
                n424 = call "Start_Initial.vi"("error in (no error)"=w374, "Reference"=w375) -> ("error out"=w367:errorcluster, "dup Reference"=w373:T5)  [unwired: 8 in]
              }
            }
            n425 = Merge Errors(w344, w343) -> (w342:errorcluster)
          }
          frame 1002 {
            # "Sequence_Pause"
            n426 = Flush Queue(queue=w390, error in (no error)=w389) -> (error out=w388:errorcluster)  [unwired: 2 out]
            n427 = call "Pause_Initial.vi"("error in (no error)"=w388, "Blinking"=TRUE, "Reference"=w394) -> ("error out"=w385:errorcluster, "dup Reference"=w393:T5)  [unwired: 7 in]
            n428 = call "write to log file.vi"("input"="!!! Pause button pressed !!!") -> ()  [unwired: 9 in, 1 out]
            n429 = local read "Current Line"() -> (w391:i32)
          }
          frame 1003 {
            # "Sequence_Stop"
            n430 = local read "Current Line"() -> (w398:i32)
            n431 = Flush Queue(queue=w405, error in (no error)=w404) -> (error out=w401:errorcluster)  [unwired: 2 out]
            n432 = property on="Sequence" class="LstBox (strict)"() -> ("Item Names"=w397:string[])  [unwired: 2 in, 2 out]
            n433 = Index Array(array=w397, index=w398) -> (element=w399:string)
            n434 = Concatenate Strings("!!! Stop button pressed !!!" ("input"), w399) -> (w400:string)
            n435 = call "write to log file.vi"("input"=w400) -> ()  [unwired: 9 in, 1 out]
            n436 = local read "Current Line"() -> (w406:i32)
            n437 = call "Program_initial.vi"("error in (no error)"=w401, "Reference"=w402) -> ("error out"=w395:errorcluster, "dup Reference"=w403:T5)  [unwired: 8 in]
          }
          frame 1004 {
            # "1. skipped sequence is added in the log\n2. Checks if it is resulted from idle or not found command."
            # "Sequence_Skip"
            n438 = local read "Current Line"() -> (w416:i32)
            n439 = Get Date/Time In Seconds() -> (seconds since 1Jan1904=w424:timestamp)
            n440 = control-ref of="Sequence"() -> (w423:refnum<vi>)
            n441 = Flush Queue(queue=w428, error in (no error)=w427) -> (queue out=w426:refnum<queue>, error out=w425:errorcluster)  [unwired: 1 out]
            n442 = property on="Sequence" class="LstBox (strict)"() -> ("Item Names"=w417:string[])  [unwired: 2 in, 2 out]
            n443 = Bundle By Name(cluster=w414, "No. of line"=w416, "Initial Time"=w424, "Sequence Ref."=w423) -> (w421:T3)
            n444 = call "Start_Initial.vi"("error in (no error)"=w425, "Reference"=w431) -> ("error out"=w429:errorcluster, "dup Reference"=w430:T5)  [unwired: 8 in]
            n445 = Unbundle By Name(w414) -> ("Status"=w412:string)
            n446 = Index Array(array=w417, index=w416) -> (element=w415:string)
            n447 = Concatenate Strings("!!! SKIP !!! " ("string"), w415) -> (w409:string)
            n448 = Equal?(x=w412, y="Unidentified command. Skipped" ("Status")) -> (x = y?=w411:bool)
            n449 = case shown="True" w411 {
              tunnel: [w432 "doo nott write to log"] -> w410
              tunnel: w409 -> [w432 _]
              frame False {
              }
              frame True {
              }
            }
            n450 = Bundle By Name(cluster=w421, "Status"=w410) -> (w420:T3)
            n451 = Unbundle By Name(w420) -> ("No. of line"=w422:i32)
            n452 = call "go_to_next_line.vi"("error in (no error)"=w429, "Message_command in"=w420, "Command Queue in"=w426) -> ("error out"=w408:errorcluster)  [unwired: 7 in, 1 out]
          }
          frame 1005 {
            # "Program Stop"
          }
          frame 1006 {
            # "Open html help document"
            n453 = call-poly <vilib>:"Open HTML Report in Browser.vi"("URL"="https://opsserver.magnet.fsu.edu/wiki/pages/j6n0H6L5/MonoVuvi_Instruction.html") -> ()  [unwired: 13 in, 2 out]
          }
          frame 1007 {
            # "1. Delete queues of command lines in the subsequences\n2. Returns to the next line of the main sequences."
            # "END SUBsequence"
            n454 = Match Pattern(string=w444, regular expression=",  line #: " ("string")) -> (before substring=w442:string)  [unwired: 1 in, 3 out]
            n455 = Get Date/Time In Seconds() -> (seconds since 1Jan1904=w463:timestamp)
            n456 = Flush Queue(queue=w466, error in (no error)=w455) -> (queue out=w458:refnum<queue>, error out=w454:errorcluster)  [unwired: 1 out]
            n457 = Unbundle By Name(w456) -> ("Sequence"=w462:refnum<vi>)
            n458 = property on="macro cmd no" class="DigNum (strict)"() -> ("Value"=w465:i32)  [unwired: 2 in, 2 out]
            n459 = local read "override command error"() -> (w451:bool)
            n460 = Increment(x=w465) -> (x+1=w464:i32)
            n461 = Bundle By Name(cluster=w452, "No. of line"=w464, "Initial Time"=w463, "Sequence Ref."=w462, "Subsequence"=string[] []) -> (w461:T3)
            n462 = call "Library2.vi"("Message_command_in"=w461, "error in (no error)"=w454) -> ("Message_command out"=w459:T4, "error out"=w447:errorcluster)  [unwired: 7 in]
            n463 = case shown="True" w451 {
              tunnel: [w467 errorcluster {"status"=FALSE, "code"=0, "source"=""} ("error in (no error)")] -> w450
              tunnel: w447 -> [w467 _]
              frame False {
              }
              frame True {
              }
            }
            n464 = Concatenate Strings("Macro Ended: " ("input"), w442) -> (w448:string)
            n465 = Enqueue Element(queue=w458, element=w459, error in (no error)=w450) -> (error out=w460:errorcluster)  [unwired: 1 in, 2 out]
            n466 = call "write to log file.vi"("input"=w448) -> ()  [unwired: 9 in, 1 out]
            n467 = call "Start_Initial.vi"("error in (no error)"=w460, "Reference"=w456) -> ("error out"=w446:errorcluster, "dup Reference"=w457:T5)  [unwired: 8 in]
            n468 = Merge Errors(w447, w446) -> (w445:errorcluster)
          }
          frame 1008 {
            # "Nested submacros are unnested to make a single expanded macro (see\ncommand line 8)."
            # "SubMacro"
            n469 = call "Start_Initial.vi"("error in (no error)"=w476, "Reference"=w477) -> ("error out"=w472:errorcluster, "dup Reference"=w475:T5)  [unwired: 8 in]
            n470 = call "RunMacro.vi"("submacro"=TRUE, "error in (no error)"=w472, "Message_command"=w473, "queue"=w474) -> ("error out"=w469:errorcluster)  [unwired: 5 in, 2 out]
          }
        }
        "Current Line" <- w71
        n471 = Unbundle By Name(w55) -> ("code"=w62:i32)
        n472 = Concatenate Strings(w51, w70) -> (→"Sequence Status":string)
        n473 = Not Equal To 0?(x=w62) -> (x != 0?=w54:bool)
        n474 = call <vilib>:"Clear Errors.vi"("error in (no error)"=w73) -> ("error out"=w57:errorcluster)  [unwired: 5 in, 1 out]
        n475 = property on="Error/\nwarning?" class="Bool (strict)"() -> ("Value"=w58:bool)  [unwired: 2 in, 2 out]
        n476 = property on="reset error indicator" class="Bool"("Visible"=w58) -> ()  [unwired: 2 in, 2 out]
        n477 = Or(x=w58, y=w54) -> (x .or. y?=w60:bool)
        n478 = Not(x="reset error indicator") -> (.not. x?=w59:bool)
        n479 = And(x=w60, y=w59) -> (x .and. y?=→"Error/\nwarning?":bool)
        n480 = case shown="True" w54 {
          tunnel: w55 -> [_ w84]
          frame False {
          }
          frame True {
            "latest error" <- w84
          }
        }
        n481 = Wait Until Next ms Multiple(millisecond multiple="wait (ms)") -> ()  [unwired: 1 out]
        "execution count" <- w64
      }
      n482 = Merge Errors(w40, w38) -> (w47:errorcluster)
    }
    frame Error {
    }
  }
  n483 = local write "sequence utility"(w10) -> ()
  n484 = Unregister For Events(event registration refnum=w21, error in=w20) -> (error out=w19:errorcluster)
  n485 = Release Queue(queue=w22, error in (no error)=w19) -> ()  [unwired: 1 in, 3 out]
  "Buffer History" <- w12
  "Buffer Edit" <- w12
